vi "WHD_VEten_0.1.5.WS_BIDIR_Inycom_baja_velocidad.vi"() -> ()   [LabVIEW 2015]
uses:
  <vilib>/LabVIEW Targets/FPGA/cRIO/shared/nicrio_ModuleControls/nicrio_cRIO-9234_DataRatesRing2.ctl
  <vilib>/RTwatchdog.llb/Watchdog expiration actions.ctl
  <vilib>/userdefined/High Color/nirio_resource_hc.ctl
  <vilib>/Platform/TimedLoop/XDataNode/timing_clust.ctl
  <vilib>/Platform/TimedLoop/XDataNode/nitl_modes.ctl
  <vilib>/Platform/TimedLoop/XDataNode/wakeup.ctl
  <vilib>/Analysis/5stat.llb/RMS (DBL).vi
  <vilib>/FPGAPlugInAG/cRIO-9031/niLvFpga_Open_cRIO-9031.vi
  <vilib>/Utility/error.llb/Error Cluster From Error Code.vi
  <vilib>/rvi/errors/niLvFpgaAdjustHostInterfaceError.vi
  <vilib>/FPGAPlugInAG/cRIO-9031/niLvFpga_Run_cRIO-9031.vi
  <vilib>/rvi/interface/common/niFpgaWaitOnOcc.vi
  <vilib>/Utility/file.llb/Write Delimited Spreadsheet (string).vi
  <vilib>/FPGAPlugInAG/cRIO-9031/niLvFpga_Reset_cRIO-9031.vi
  <vilib>/measure/madcrms.llb/Basic Averaged DC-RMS for 1 Chan.vi
  <vilib>/measure/maspectr.llb/FFT Spectrum (Mag-Phase) for 1 Chan.vi
  <vilib>/Utility/config.llb/Write Key (Double).vi
  <vilib>/FPGAPlugInAG/cRIO-9031/niLvFpga_Close_cRIO-9031.vi
  <vilib>/rvi/interface/nirviOpenFPGA/nirviOpenFPGA.xnode
  FPGA Bitfiles/WRDArabia_FPGATarget_FPGA8a2wsBIdirec_ph5KjwleieA.lvbitx
  <vilib>/rvi/interface/nirviReadWriteControl/nirviReadWriteControl.xnode
  <vilib>/rvi/interface/nirviMethod/nirviMethod.xnode
  <vilib>/platform/TimedLoop/XDataNode/XDataNode.xnode
  <vilib>/rvi/interface/nirviCloseFPGA/nirviCloseFPGA.xnode
  <vilib>/NI_Real-Time Target Support.lvlib
  <vilib>/rvi/errors/niLvFpgaMergeErrorWithErrorCode.vi
  AURA_Wheel/Json2Labv.lvlib
  AURA_Wheel/AuraWheelAPI/AuraWheel.lvlib
  NiFpgaLv.dll
  <vilib>/FPGAPlugInAG/cRIO-9031/niLvFpga_ConfigureFifo_cRIO-9031.vi
  <vilib>/FPGAPlugInAG/cRIO-9031/niLvFpga_StartFifo_cRIO-9031.vi
  <vilib>/FPGAPlugInAG/cRIO-9031/niLvFpga_ReadFifo_cRIO-9031.vi
  <vilib>/FPGAPlugInAG/cRIO-9031/niLvFpga_StopFifo_cRIO-9031.vi
  <vilib>/measure/NI_MAPro.lvlib
  <vilib>/Analysis/NI_AALPro.lvlib
  <vilib>/Analysis/NI_AALBase.lvlib
  <vilib>/Utility/config.llb/NI_LVConfig.lvlib
  <vilib>/Platform/TimedLoop/XDataNode/XDNodeRunTimeDep.lvlib
  Library/IF2_Reader/IF2_Reader.lvlib
panel:
  out "size(s) 2":i32[](array[numeric])
  out "freq_cutlow":dbl
  out "freq_cuthigh":dbl
  out "Radios_por_ejes":dbl[](array[numeric])
  out "Radios ruedas":dbl[](array[numeric])
  out "Frequency":dbl[](array[numeric])
  out "Value to compare":dbl[](array[numeric])
  in  "Developer password":string
  out "Waveform Graph":waveform(sgl)[](graph)
  out "min":dbl[](array[numeric])
  out "max":dbl[](array[numeric])
  out "median":dbl[](array[numeric])
  out "mean":dbl[](array[numeric])
  in  "Accelerometer":i32
  out "Low cutoff freq":dbl
  out "noise_range":dbl
  out "Numeric":i32
  out "Calibration parameter":dbl
  out "Accel.detected":i32
  out "Mean\nfrequency":dbl format="%0.2f"
  out "Nº meas":i32
  out "Array":i32[](array[numeric])
  out "sorted array":i32[](array[numeric])
  out "Array 3":i32[](array[numeric])
  out "max value":i32
  out "max index(es)":i32
  out "element":i32
  out "size(s) 3":i32
  out "size(s)":i32[](array[numeric])
  out "Valid\nindex":i32[](array[numeric])
  out "Acquiring time":dbl
  out "Inicio pasada 2":timestamp
  out "calibration log":path
  out "date/time string 2":string
  out "Folder":path
  in  "Developer commad":string
  out "Save calibration":bool
  out "Pattern amplitude (g)":dbl=1.02
  out "Pattern frequency (Hz)":dbl=159.2
  out "Report":string
  out "AURA wheel test":bool
  out "LOG.txt":path
  out "Report_AURA":string
  out "error FPGA":errorcluster
  out "error AURA":errorcluster
  out "error manipulacion archivos":errorcluster
  out "Response headers":string
  out "Max RMS Ruedas":dbl[][](array[numeric])
  out "TAGs LR6":string[](array[string])
  out "TAGs HEX":string[](array[string])
  out "Parar":bool
  out "result":bool
  out "TAGs":string[](array[string])
  out "Temperatura (ºC)":dbl
  out "V (m/s)":dbl
  out "Digital?":bool=TRUE
  out "Watchdog config":T1={"reset"=FALSE, "occurrence"=FALSE, "trigger protocol"=enum."active high", "trigger line"=enum."none", "disable watchdog on VI exit"=TRUE}
  out "Tiempo de adquisicion":dbl=10.0
  out "Adquirir":bool
  out "Nº Ruedas 1":i32
  out "NºRuedas 2":i32
  out "Disco Duro Disponible (bytes)":i64
  out "Buffer Overflow":bool
  out "Buffer Underflow":bool
  out "Archivo\nvalido?":bool
  out "Número de ejes detectados":i32
  out "Ejes_convoy":i32
  out "Tiempo de paso (s)":dbl
  out "created path":path
  out "Nombre de archivo":path[](array[path])
  out "LR6 IP address":string="192.168.106.94"
  out "Port LR6":u16=2001
  out "T fuera rango":bool
  out "Frecuencia de muestreo (Hz)":dbl=25600.0
  out "Escaneos de la FIFO por canal":u32=5000
  out "Tiempo extra al detector de paso (s)":dbl=1.0
  out "dt RMS":dbl=256.0
  out "Frecuencia de muestreo y módulo CRIO":T2=2 items=["51.200 kS/s (NI 9234)"=1, "25.600 kS/s (NI 9234)"=2, "17.067 kS/s (NI 9234)"=3, "12.800 kS/s (NI 9234)"=4, "10.240 kS/s (NI 9234)"=5, "8.533 kS/s (NI 9234)"=6, "7.314 kS/s (NI 9234)"=7, "6.400 kS/s (NI 9234)"=8, "5.689 kS/s (NI 9234)"=9, "5.120 kS/s (NI 9234)"=10, "4.654 kS/s (NI 9234)"=11, "4.267 kS/s (NI 9234)"=12, "3.938 kS/s (NI 9234)"=13, "3.657 kS/s (NI 9234)"=14, "3.413 kS/s (NI 9234)"=15, "3.200 kS/s (NI 9234)"=16, "3.012 kS/s (NI 9234)"=17, "2.845 kS/s (NI 9234)"=18, "2.695 kS/s (NI 9234)"=19, "2.560 kS/s (NI 9234)"=20, "2.438 kS/s (NI 9234)"=21, "2.328 kS/s (NI 9234)"=22, "2.226 kS/s (NI 9234)"=23, "2.133 kS/s (NI 9234)"=24, "2.048 kS/s (NI 9234)"=25, "1.969 kS/s (NI 9234)"=26, "1.896 kS/s (NI 9234)"=27, "1.829 kS/s (NI 9234)"=28, "1.765 kS/s (NI 9234)"=29, "1.707 kS/s (NI 9234)"=30, "1.652 kS/s (NI 9234)"=31]
  out "Puerto RFID":u16=2189
  out "IP RFID":string="192.168.106.99"
  out "Offset_rueda WS 2":fxp<+/-,24,-4>=0.004999998956918716 format="%.27g"
  out "Count(mSec)":u32=2
  out "RFID NEM on?":bool
  out "RFID LR6 on?":bool
  out "Canal cero WS1?":bool
  out "Canal cero WS2":bool
  in  "Calibration":bool
  out "Direccion 0?":bool
  out "Boton Adquirir?":bool
  out "RuedaDetectada2?":bool=TRUE
  out "RuedaDetectada1?":bool=TRUE
  out "Timeout ruedas":dbl
  out "Borrar archivos\nadquisicion con error":bool
  out "Able watchdog?":bool
  out "Reset watchdog?":bool
  out "Leer config RFID NEM":bool
  out "bytes to read":i32
  out "DeviceAddress":u8
  out "timeout ms (60000)":i32
  out "Max archivos":u32=2
  out "Bytes libre despues de borrar":u32=2
  out "Bytes min libre":u32=2
  out "Nº de acelerómetros":i32
  out "Nº inductivos":i32
  out "Offset_rueda WS 1":fxp<+/-,24,-4>=0.004999998956918716 format="%.27g"
  out "TAGs_AURAwheel":string[][](array[string])
  out "Plataformas?":bool
  out "Nº Ejes":i32[](array[numeric])
  out "Nº UTs":i32
  out "it-read-LR6":i32[](array[numeric])
  out "it-LR6":i32
  out "RFID_LR6_Error":errorcluster
  out "Series_flota":string[](array[string])
  out "Tabla_flota":string[][](array[string])
  out "Puntos medios de las ventanas":dbl[][](array[numeric])
  out "configuration file path":path=path "c:/Parametros.cfg"
  out "IP synchr":string
  out "data":cluster{"status":string}
  out "confRFID":path=path "c:/RFID/TAGS.csv"
  out "TAGS leidos":path=path "c:/RFID/TAGS.csv"
  out "Use Aura?":bool
  out "Parametros AuraWheel":string[](array[string])
  out "Parámetros acelerómetros":dbl[](array[numeric])
  out "Fin":bool
  out "Contador":i32=1
  out "Path LOG":path=path "c:/TEST"
  out "Fallo fotocelula":bool
  out "Path_Borrar":path=path "c:/Trenes"
  out "Longitud de la unidad":dbl
  out "Aviso no detección":string
  out "Time to Acquire Block (ms)":i32
  out "Distancia de acelerómetros":dbl[](array[numeric])
  out "Block Size":u32
  out "Distancias generales":dbl[](array[numeric])
  out "Reset del controlador":bool
  out "Parar la aplicación":bool
  out "date/time string":string
  out "Timeout ruedas":bool
  out "Tiempo":dbl
  out "Inicio pasada":timestamp
  out "Ultimo TEST":timestamp
  out "Fuente":bool=TRUE
  out "DC OK":string
  out "Aviso temperatura":string
  out "connection ID":refnum<k5>
  # "Calibration - Noise analysis"
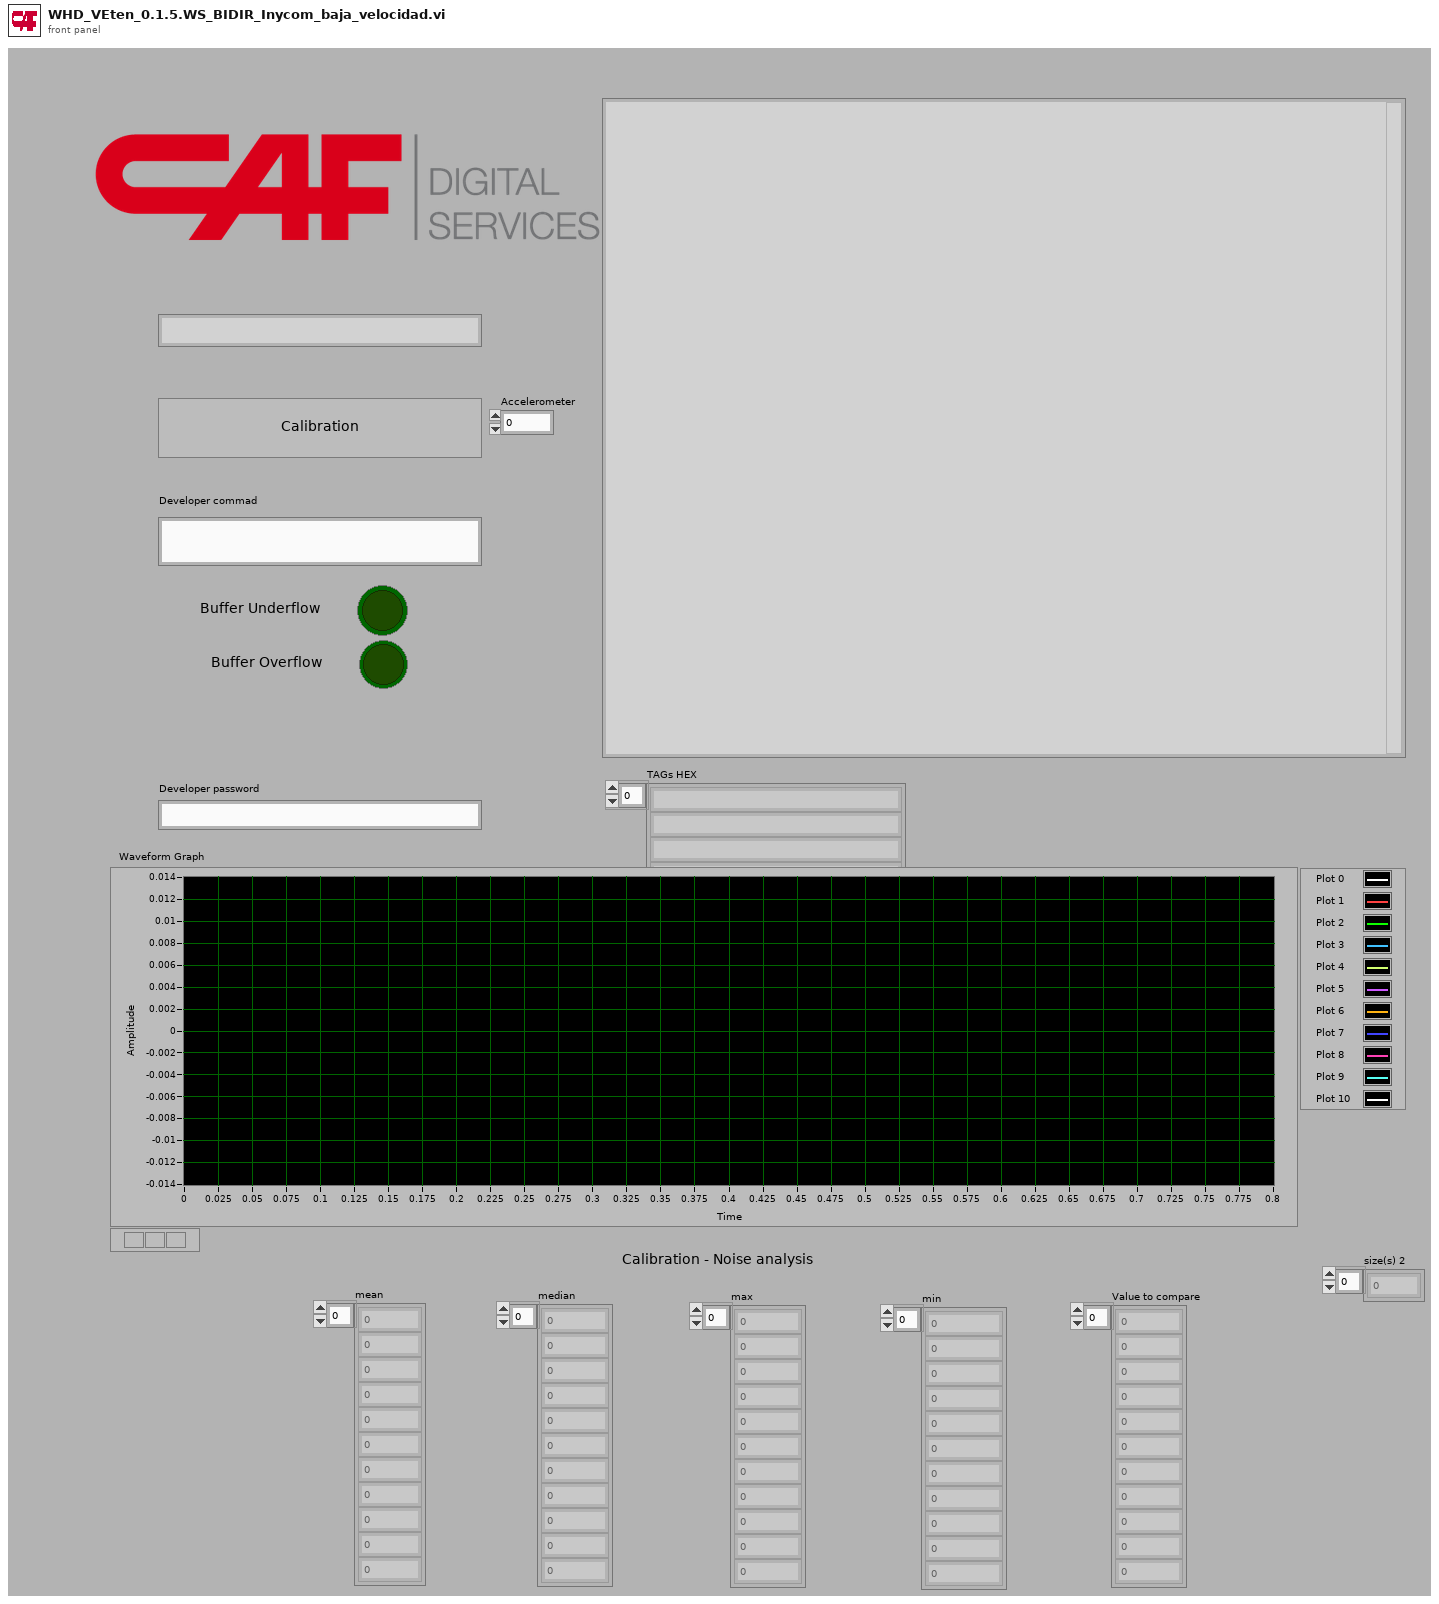
[diagram p1: front panel]
types:
  T1 = typedef "Watchdog expiration actions.ctl" = cluster{"reset":bool, "occurrence":bool, "trigger protocol":enum16{"active high", "active low", "open collector"}, "trigger line":enum16{"none", "line 0", "line 1", "line 2", "line 3", "line 4", "line 5", "line 6", "line 7", "SMB line 0"}, "disable watchdog on VI exit":bool}
  T2 = typedef "nicrio_cRIO-9234_DataRatesRing2.ctl" = u8
  T3 = typedef "nirio_resource_hc.ctl" = tag
  T4 = enum16{"open", "replace", "create", "open or create", "replace or create", "replace or create with confirmation"}
  T5 = enum16{"big-endian, network order", "native, host order", "little-endian"}
  T6 = typedef "XDNodeRunTimeDep.lvlib/timing_clust.ctl" = cluster{"Expected End [f-1]":u64, "Actual End [f-1]":u64, "Finished Late? [f-1]":bool, "Expected End [i-1]":u64, "Actual End [i-1]":u64, "Finished Late? [i-1]":bool, "Expected Start [i]":u64, "Actual Start [i]":u64, "Expected Start [f]":u64, "Actual Start [f]":u64, "Source Name":string, "Structure Name":string, "Period":i64, "Deadline":i64, "Offset":i64, "Start":i64, "Priority":i32, "Timeout":i32, "Mode":T7, "Wakeup Reason":T8, "Error":errorcluster, "Source Type":string, "Secondary Source Type":string, "Global End Time":u64, "Global Start Time":u64, "Frame Duration":u64, "Iteration Duration":u64, "Assigned CPU":i32, "I/O Scan Engine Mode":u32}
  T7 = typedef "XDNodeRunTimeDep.lvlib/nitl_modes.ctl" = enum32{"No Change", "Process missed periods, maintain original phase", "Discard missed periods, maintain original phase", "Process missed periods, ignore original phase", "Discard missed periods, ignore original phase"}
  T8 = typedef "XDNodeRunTimeDep.lvlib/wakeup.ctl" = enum32{"Normal", "Aborted", "Asynchronous wakeup", "Timing source error", "Timed loop error", "Timeout"}
  T9 = cluster{"error IO":errorcluster, bool[], u32[], string[], dbl[]}
  T10 = cluster{"error out":errorcluster, dbl[], "TagArray":string[], "Direccion 0?":bool}
  T11 = cluster{"g_ts":dbl, "p_sp":dbl, "p_tp":dbl, "p_tg":cluster{"tg_n":dbl, "tg_t":string}[], "p_ax":cluster{"ax_n":dbl, "ax_sp":dbl, "ax_wh":cluster{"wh_p":dbl, "wh_a1":dbl, "wh_a2":dbl, "wh_a3":dbl, "wh_a4":dbl}[], "ax_fq":cluster{"wh_p":dbl, "wh_a1":dbl, "wh_a2":dbl, "wh_a3":dbl, "wh_a4":dbl}[], "ax_amp":cluster{"wh_p":dbl, "wh_a1":dbl, "wh_a2":dbl, "wh_a3":dbl, "wh_a4":dbl}[], "ax_en":cluster{"wh_p":dbl, "wh_a1":dbl, "wh_a2":dbl, "wh_a3":dbl, "wh_a4":dbl}[]}[]}
  T12 = typedef "NI_LVConfig.lvlib/Config Data RefNum.ctl" = refnum<k1>
  T13 = cluster{"IP":string, "Port":u16, "ReaderConfigFile":path, "ROspecConfigFile":path}
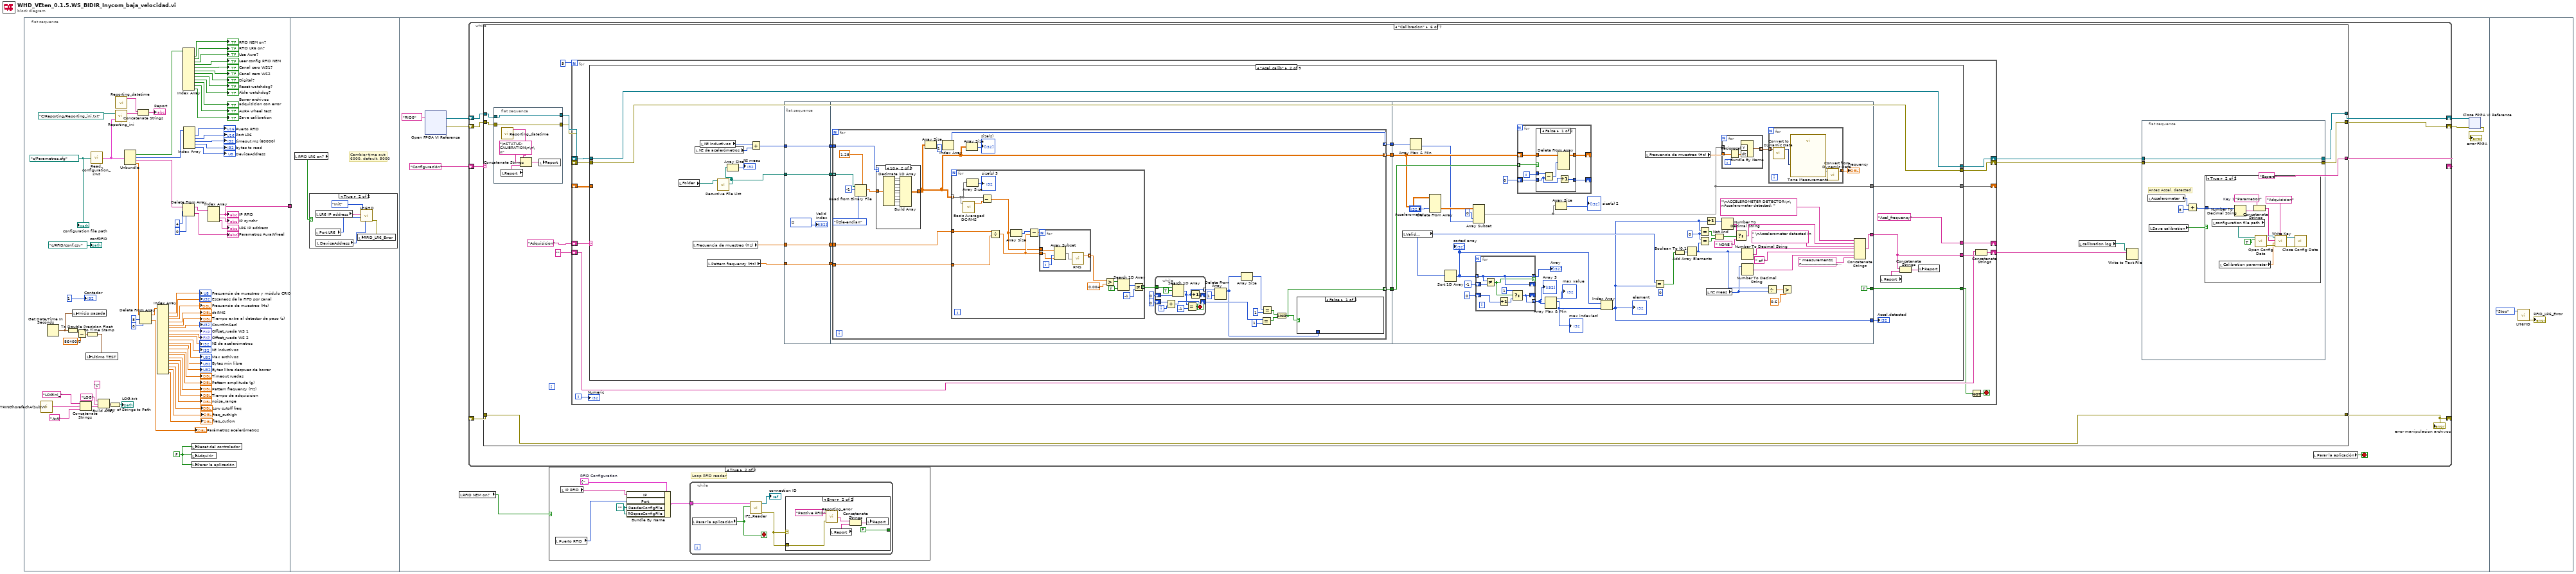
[diagram p0: block diagram]
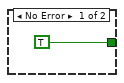
[diagram p4: hidden frame]
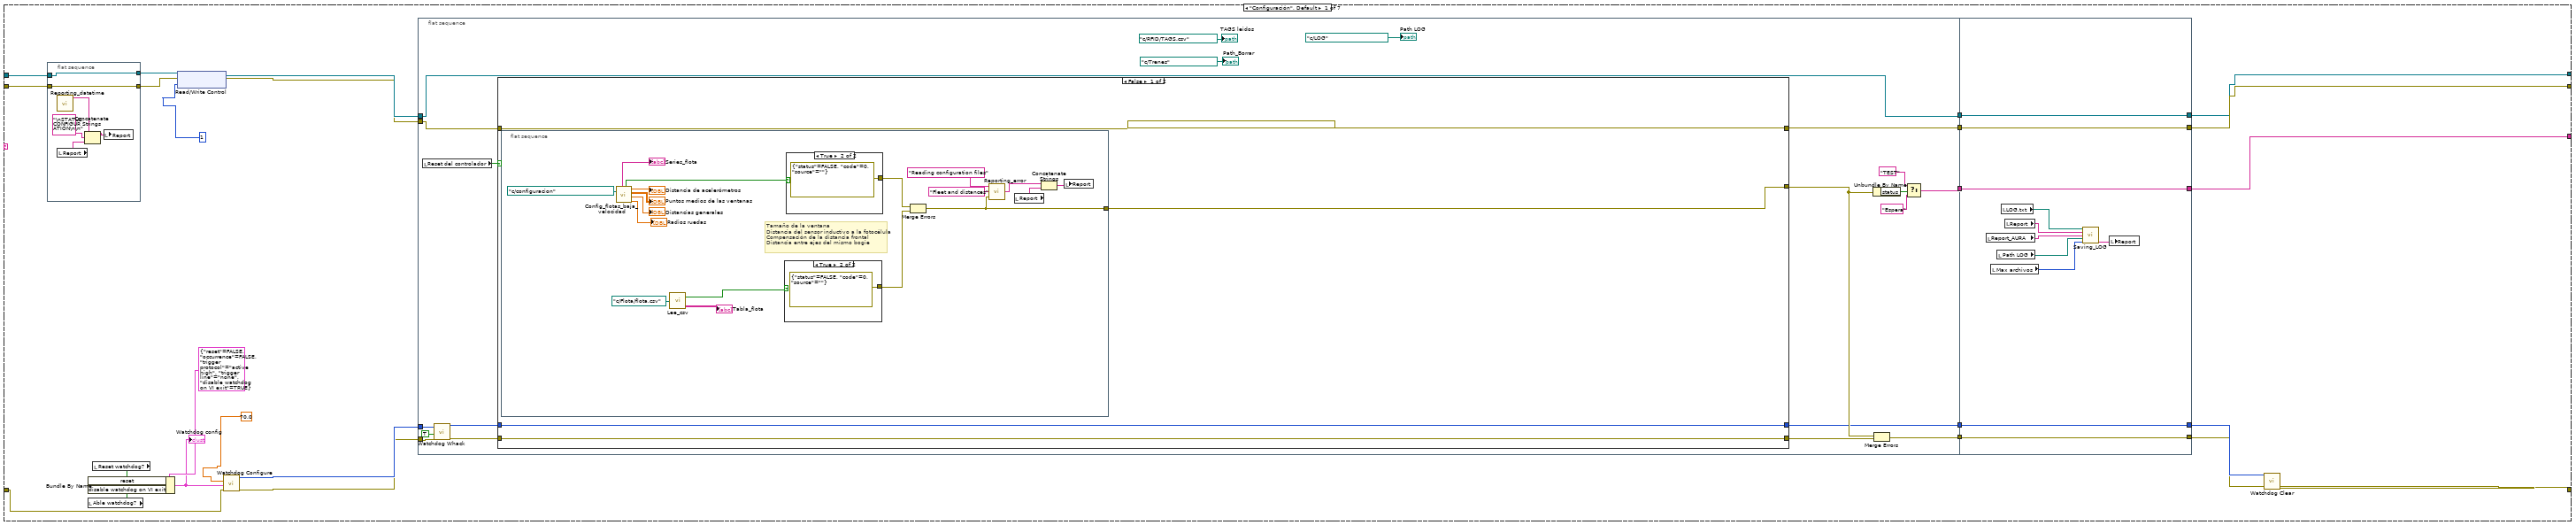
[diagram p5: hidden frame]
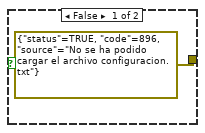
[diagram p6: hidden frame]
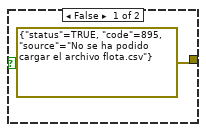
[diagram p7: hidden frame]
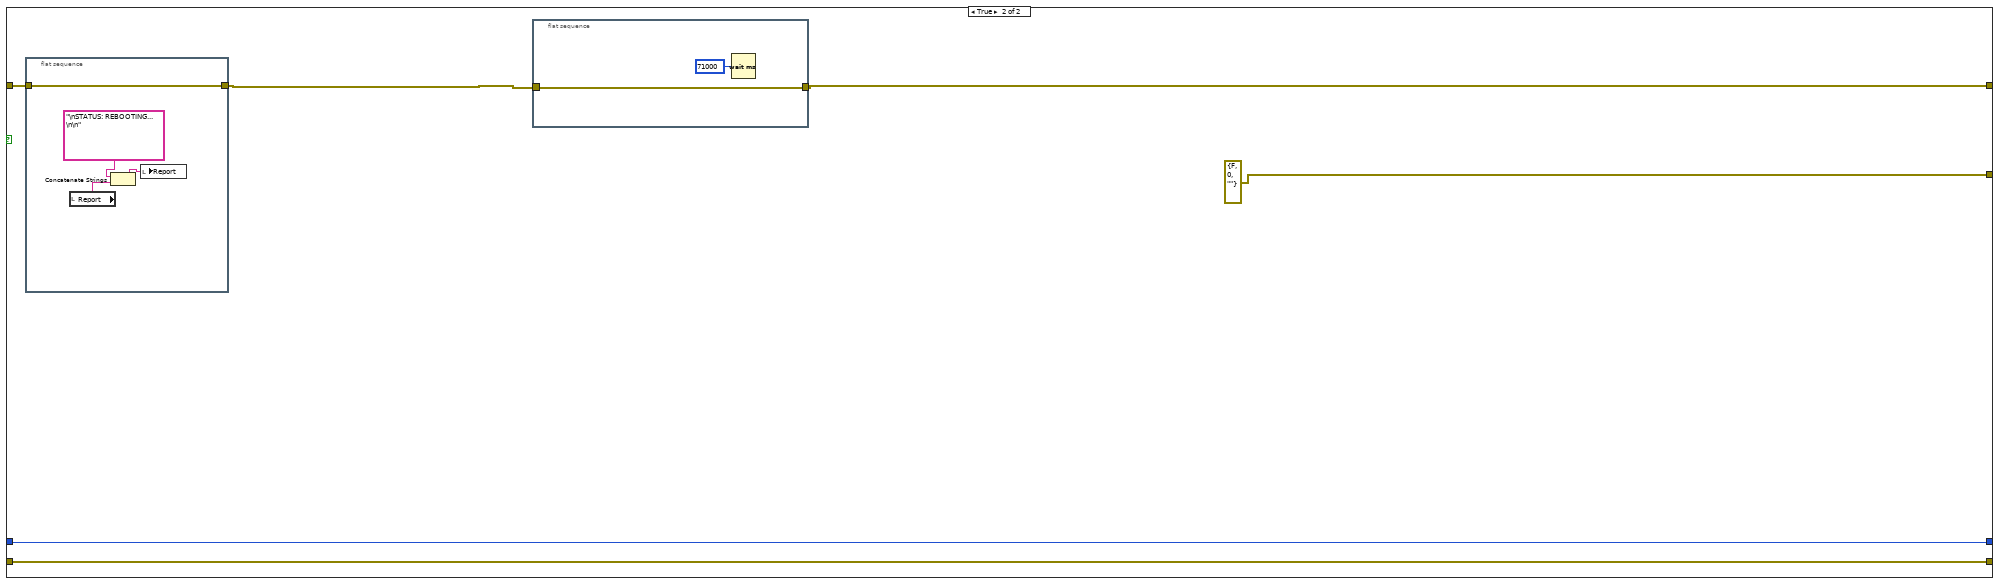
[diagram p8: hidden frame]
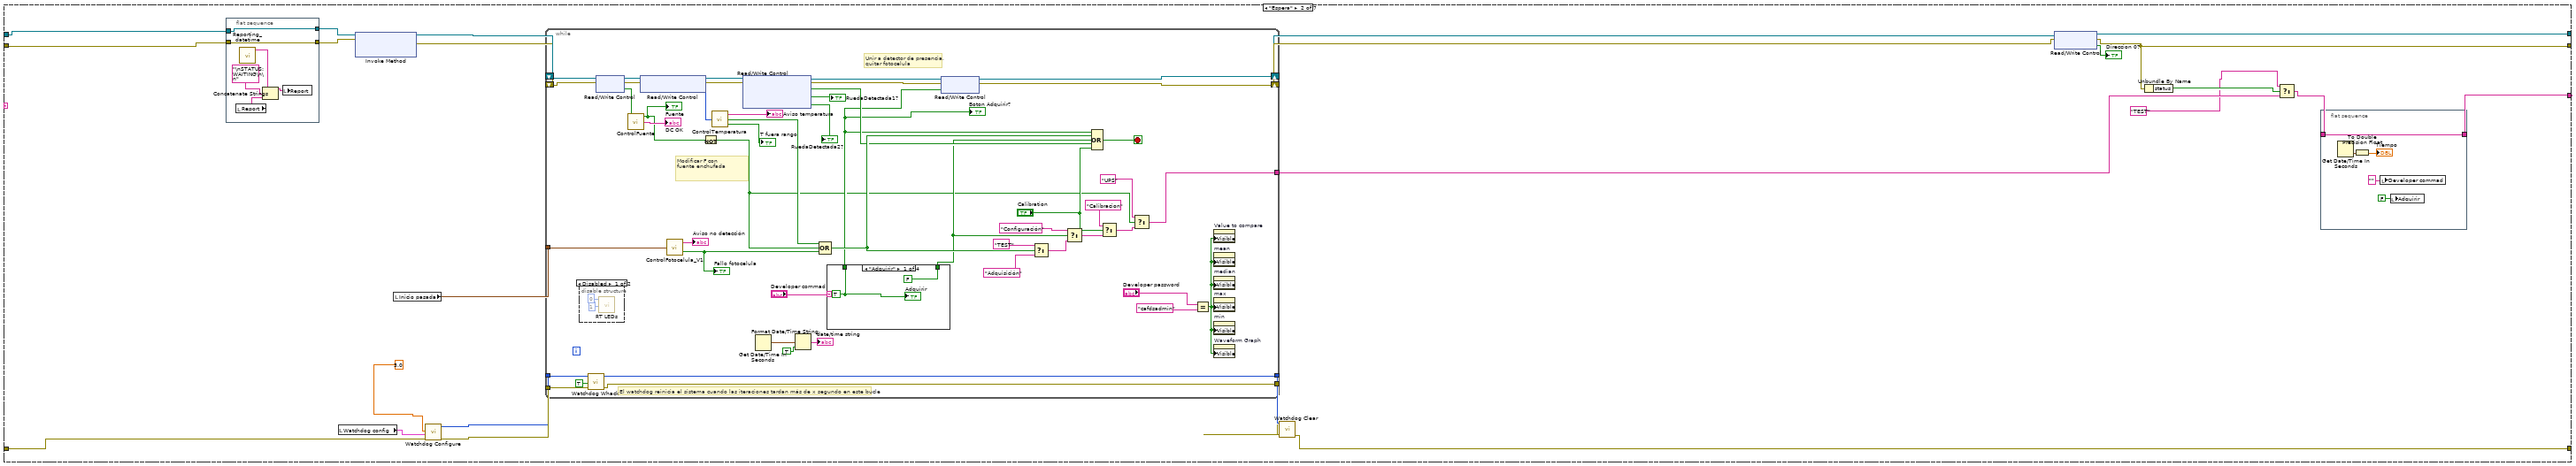
[diagram p9: hidden frame]
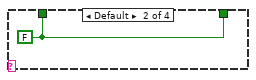
[diagram p10: hidden frame]
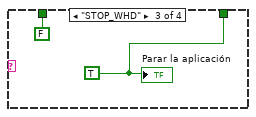
[diagram p11: hidden frame]
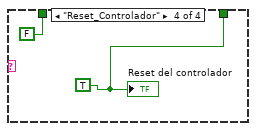
[diagram p12: hidden frame]
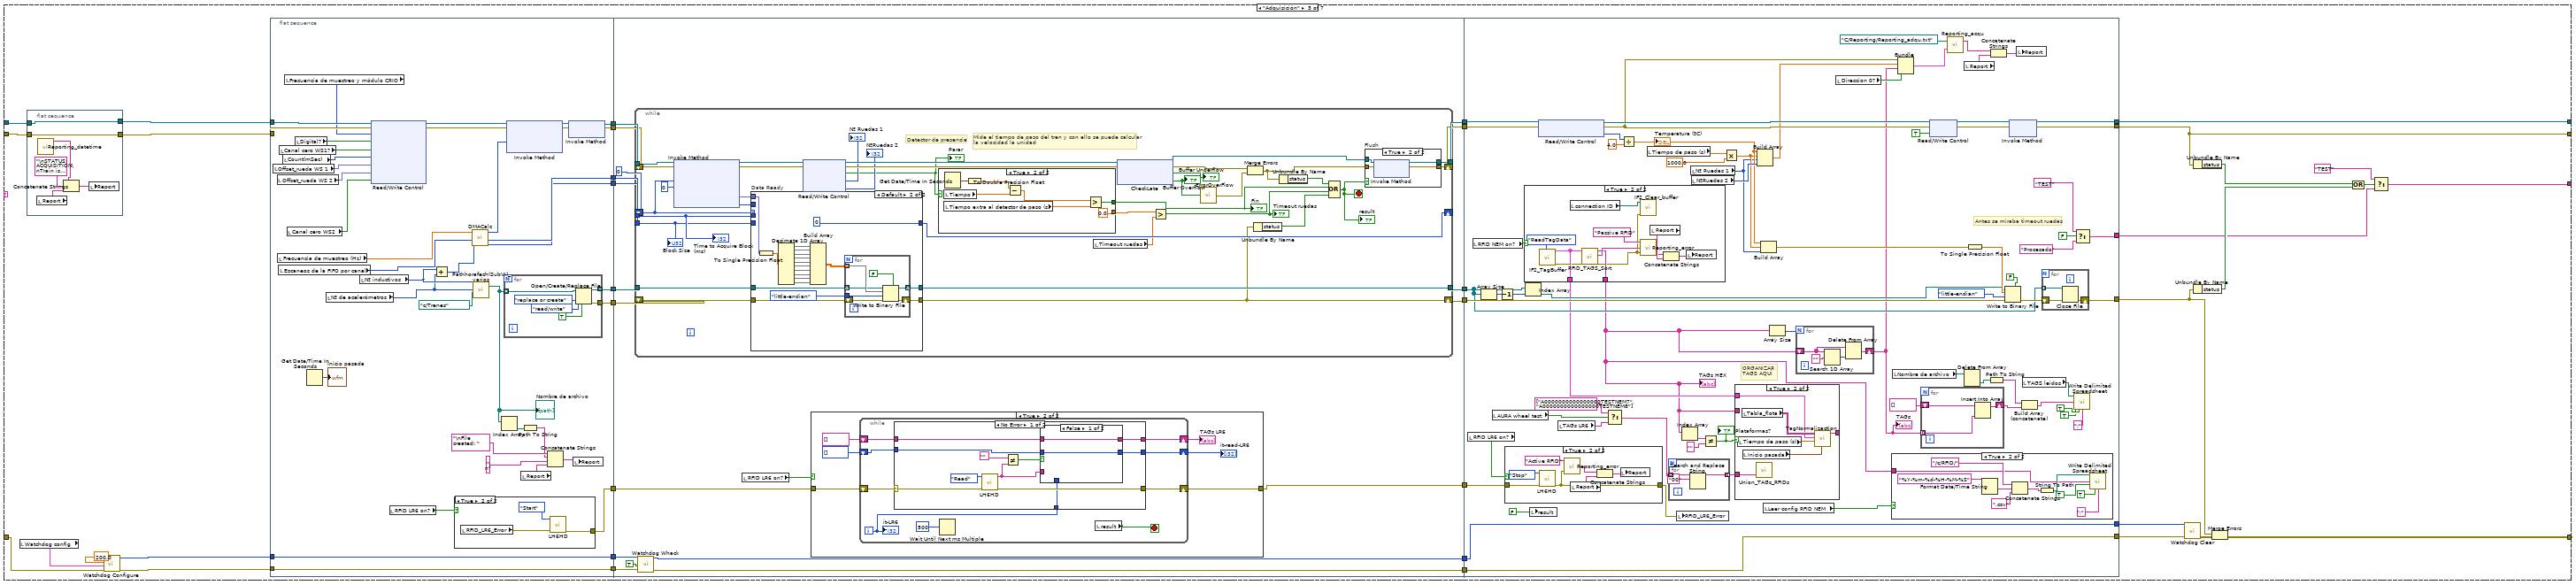
[diagram p14: hidden frame]
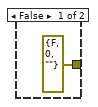
[diagram p15: hidden frame]
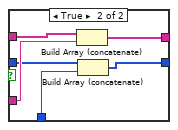
[diagram p17: hidden frame]
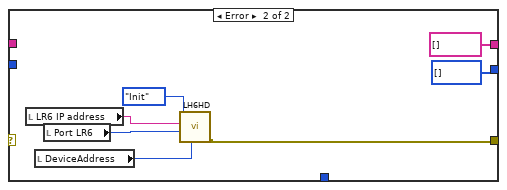
[diagram p18: hidden frame]
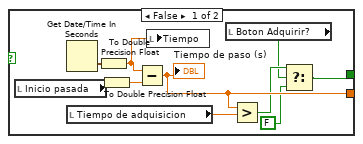
[diagram p19: hidden frame]
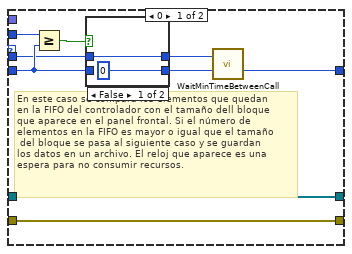
[diagram p20: hidden frame]
diagram:
  n1 = flat-sequence {
    tunnel: [w6] -> w1
    tunnel: w1 -> [_]
    frame #0 {
      w7 = FALSE ("Reset del controlador")
      w68 = path "c:/Parametros.cfg" ("configuration file path")
      n2 = call "STRINGhorafechA(SubVI).vi"() -> ("STRINGhora_fecha"=w18:string)
      n3 = Get Date/Time In Seconds() -> (seconds since 1Jan1904=w73:timestamp)
      n4 = To Double Precision Float(number=w73) -> (double precision float=w75:dbl)
      n5 = local write "Inicio pasada"(w73) -> ()
      n6 = Subtract(x=w75, y=86400.0) -> (x-y=w74:dbl)
      n7 = Concatenate Strings("LOGini_" ("string"), w18, ".txt" ("string")) -> (w20:string)
      n8 = To Time Stamp(1:w74) -> (0:w72:timestamp)
      n9 = local write "Ultimo TEST"(w72) -> ()
      n10 = call "Read_configuration_2ws.vi"("configuration file path"=w68) -> ("output cluster"=w24:T9)
      n11 = Build Array("c", "LOG" ("element"), w20) -> (w17:string[])
      n12 = Array of Strings to Path(0:w17) -> (2:→"LOG.txt":path)  [unwired: 1 out]
      n13 = call "Reporting_ini.vi"("Configuration cluster"=w24, "address repoting"=path "C:/Reporting/Reporting_ini.txt" ("file (use dialog)")) -> ("Reporting"=w23:string)  [unwired: 1 in]
      n14 = call "Reporting_datetime.vi"() -> ("String"=w21:string)  [unwired: 11 in]
      n15 = Unbundle(w24) -> (w71:bool[], w70:u32[], w63:string[], w67:dbl[])  [unwired: 1 out]
      n16 = Concatenate Strings(w21, w23) -> (→"Report":string)
      n17 = Delete From Array(array=w67, length=8, index=8) -> (deleted portion=→"Parámetros acelerómetros":dbl[], array with subset deleted=w66:dbl[])
      n18 = Index Array(array=w66) -> (element #1=→"Frecuencia de muestreo y módulo CRIO":dbl, element #2=→"Escaneos de la FIFO por canal":dbl, element #3=→"Frecuencia de muestreo (Hz)":dbl, element #4=→"dt RMS":dbl, element #5=→"Tiempo extra al detector de paso (s)":dbl, element #6=→"Count(mSec)":dbl, element #7=→"Offset_rueda WS 1":dbl, element #8=→"Offset_rueda WS 2":dbl, element #9=→"Nº de acelerómetros":dbl, element #10=→"Nº inductivos":dbl, element #11=→"Max archivos":dbl, element #12=→"Bytes min libre":dbl, element #13=→"Bytes libre despues de borrar":dbl, element #14=→"Timeout ruedas":dbl, element #15=→"Pattern amplitude (g)":dbl, element #16=→"Pattern frequency (Hz)":dbl, element #17=→"Tiempo de adquisicion":dbl, element #18=→"noise_range":dbl, element #19=→"Low cutoff freq":dbl, element #20=→"freq_cuthigh":dbl, element #21=→"freq_cutlow":dbl)  [unwired: 21 in]
      n19 = Index Array(array=w71) -> (element #1=→"RFID NEM on?":bool, element #2=→"RFID LR6 on?":bool, element #3=→"Use Aura?":bool, element #4=→"Leer config RFID NEM":bool, element #5=→"Canal cero WS1?":bool, element #6=→"Canal cero WS2":bool, element #7=→"Digital?":bool, element #8=→"Reset watchdog?":bool, element #9=→"Able watchdog?":bool, element #10=→"Borrar archivos\nadquisicion con error":bool, element #11=→"AURA wheel test":bool, element #12=→"Save calibration":bool)  [unwired: 12 in]
      n20 = Delete From Array(array=w63, length=4, index=0) -> (deleted portion=→"Parametros AuraWheel":string[], array with subset deleted=w62:string[])
      n21 = Index Array(array=w70) -> (element #1=→"Puerto RFID":u32, element #2=→"Port LR6":u32, element #3=→"timeout ms (60000)":u32, element #4=→"bytes to read":u32, element #5=→"DeviceAddress":u32)  [unwired: 5 in]
      n22 = local write "Reset del controlador"(w7) -> ()
      n23 = local write "Adquirir"(w7) -> ()
      n24 = local write "Parar la aplicación"(w7) -> ()
      n25 = Index Array(array=w62) -> (element #1=w6:string, element #2=→"IP synchr":string, element #3=→"LR6 IP address":string)  [unwired: 3 in]
      "IP RFID" <- w6
      "Contador" <- 1
      "confRFID" <- path "c:/RFID/conf.csv" ("file path (use dialog)")
      "configuration file path" <- w68
    }
    frame #1 {
      # "Cambiar time out:\n6000, default, 5000"
      n26 = local read "RFID LR6 on?"() -> (w77:bool)
      n27 = case shown="True" w77 {
        frame False {
        }
        frame True {
          n28 = local read "LR6 IP address"() -> (w78:string)
          n29 = local read "Port LR6"() -> (w79:u16)
          n30 = local read "DeviceAddress"() -> (w80:u8)
          n31 = call "LH6HD.vi"("DeviceAddress"=w80, "Reader Port"=w79, "IP Address"=w78, "Action"=enum16{"Init", "Start", "Read", "Stop", "Exit"}."Init") -> ("error out"=w82:errorcluster)  [unwired: 6 in, 1 out]
          n32 = local write "RFID_LR6_Error"(w82) -> ()
        }
      }
    }
    frame #2 {
      n33 = xnode "Open FPGA VI Reference"("resource name"=T3 "RIO0") -> ("FPGA VI Reference Out"=w90:refnum<k20>, "error out"=w89:errorcluster)  [unwired: 1 in]
      n34 = local read "RFID NEM on?"() -> (w83:bool)
      n35 = while {
        shift-right: [w107] -> _
        shift-left: "Configuración" -> [w115]
        shift-right: [w109] -> w86
        shift-left: w90 -> [w114]
        shift-right: [w108] -> w85
        shift-left: w89 -> [w113]
        shift-right: [w112] -> _
        shift-left: _ -> [w111]
        stop <- w110 stop-if-true
        n36 = case shown="\"Calibracion\"" w115 {
          tunnel: [w130 w234 w329 w695 w983 "Espera" "Espera" ("t")] -> w107
          tunnel: [w140 w222 w343 w684 w982 w1049 w1843] -> w109
          tunnel: [w141 w221 w344 w682 w981 w1047 w1842] -> w108
          tunnel: w114 -> [w124 w220 w315 w685 w982 w1060 w1837]
          tunnel: w113 -> [w123 w219 w314 w683 w974 w1059 w1839]
          tunnel: [w137 w228 w341 w680 w973 w1048 w1840] -> w112
          tunnel: w111 -> [w129 w233 w325 w694 w970 w1048 w1840]
          frame "Configuración", Default {
            n37 = flat-sequence {
              tunnel: w124 -> [w147]
              tunnel: w123 -> [w146]
              tunnel: [w147] -> w122
              tunnel: [w146] -> w121
              frame #0 {
                n38 = call "Reporting_datetime.vi"() -> ("String"=w142:string)  [unwired: 11 in]
                n39 = local read "Report"() -> (w143:string)
                n40 = Concatenate Strings(w142, "\nSTATUS: CONFIGURATION\n\n", w143) -> (w145:string)
                n41 = local write "Report"(w145) -> ()
              }
            }
            n42 = local read "Able watchdog?"() -> (w134:bool)
            n43 = local read "Reset watchdog?"() -> (w135:bool)
            n44 = Bundle By Name(cluster=T1 {"reset"=FALSE, "occurrence"=FALSE, "trigger protocol"=enum."active high", "trigger line"=enum."none", "disable watchdog on VI exit"=TRUE} ("expiration actions"), "reset"=w135, "disable watchdog on VI exit"=w134) -> (w128:T1)
            "Watchdog config" <- w128
            n45 = xnode "Read/Write Control"("FPGA VI Reference In"=w122, "error in"=w121, "Cycles to Filter"=u16 1) -> ("FPGA VI Reference Out"=w133:refnum<k20>, "error out"=w132:errorcluster)
            n46 = call <vilib>:"Watchdog Configure.vi"("error in (no error)"=w129, "expiration actions"=w128, "timeout (1 sec)"=70.0) -> ("error out"=w125:errorcluster, "watchdogID"=w126:u64)  [unwired: 1 in, 2 out]
            n47 = flat-sequence {
              tunnel: w133 -> [w159]
              tunnel: w132 -> [w156]
              tunnel: w126 -> [w149]
              tunnel: w125 -> [w148]
              tunnel: [w158] -> w120
              tunnel: [w166] -> w119
              tunnel: [w159] -> w118
              tunnel: [w161] -> w117
              tunnel: [w153] -> w116
              tunnel: [w212] -> w139
              tunnel: [w213] -> w138
              tunnel: [w214] -> w140
              tunnel: [w215] -> w130
              tunnel: [w216] -> w141
              tunnel: w120 -> [w216]
              tunnel: w119 -> [w215]
              tunnel: w118 -> [w214]
              tunnel: w117 -> [w213]
              tunnel: w116 -> [w212]
              frame #0 {
                n48 = local read "Reset del controlador"() -> (w155:bool)
                n49 = call <vilib>:"Watchdog Whack.vi"("error in (no error)"=w148, "reset watchdog after expire? (F)"=TRUE, "watchdogID in"=w149) -> ("error out"=w151:errorcluster, "watchdogID out"=w152:u64)  [unwired: 2 in, 1 out]
                n50 = case shown="False" w155 {
                  tunnel: w156 -> [w171 w195]
                  tunnel: [w171 w198] -> w158
                  tunnel: [w168 errorcluster {"status"=FALSE, "code"=0, "source"=""} ("error IO")] -> w157
                  tunnel: [w170 w197] -> w153
                  tunnel: w152 -> [w170 w197]
                  tunnel: w151 -> [w169 w196]
                  tunnel: [w169 w196] -> w150
                  frame False {
                    n51 = flat-sequence {
                      tunnel: [w179] -> w168
                      frame #0 {
                        # "Tamaño de la ventana\nDistancia del sensor inductivo a la fotocélula\nCompensación de la distancia frontal\nDistancia entre ejes del mismo bogie"
                        n52 = call "Config_flotas_baja_velocidad.vi"("file path (dialog if empty)"=path "c:/configuracion") -> ("Radios ruedas"=→"Radios ruedas":dbl[], "Distancias generales"=→"Distancias generales":dbl[], "Puntos medios de las ventanas"=→"Puntos medios de las ventanas":dbl[][], "Distancia de acelerómetros"=→"Distancia de acelerómetros":dbl[], "Distacias y medidas de dispositivos"=w176:bool, "Series_flota"=→"Series_flota":string[])  [unwired: 5 in]
                        n53 = call "Lee_csv.vi"("Path"=path "c:/Flota/flota.csv") -> ("Tabla_flota"=→"Tabla_flota":string[][], "Lectura_OK?"=w187:bool)
                        n54 = case shown="True" w187 {
                          tunnel: [errorcluster {"status"=TRUE, "code"=895, "source"="No se ha podido cargar el archivo flota.csv"} ("error out") errorcluster {"status"=FALSE, "code"=0, "source"=""} ("error out")] -> w188
                          frame False {
                          }
                          frame True {
                          }
                        }
                        n55 = case shown="True" w176 {
                          tunnel: [errorcluster {"status"=TRUE, "code"=896, "source"="No se ha podido cargar el archivo configuracion.txt"} ("error out") errorcluster {"status"=FALSE, "code"=0, "source"=""} ("error out")] -> w189
                          frame False {
                          }
                          frame True {
                          }
                        }
                        n56 = Merge Errors(w189, w188) -> (w179:errorcluster)
                        n57 = call "Reporting_error.vi"("error out 2"=w179, "Concept explanation"="Fleet and distances", "Concept"="Reading configuration files") -> ("Reporting"=w181:string)
                        n58 = local read "Report"() -> (w180:string)
                        n59 = Concatenate Strings(w181, w180) -> (w182:string)
                        n60 = local write "Report"(w182) -> ()
                      }
                    }
                  }
                  frame True {
                    n61 = flat-sequence {
                      tunnel: w195 -> [w203]
                      tunnel: [w203] -> w194
                      frame #0 {
                        n62 = local read "Report"() -> (w202:string)
                        n63 = Concatenate Strings("\nSTATUS: REBOOTING...\n\n", w202) -> (w200:string)
                        n64 = local write "Report"(w200) -> ()
                      }
                    }
                    n65 = flat-sequence {
                      tunnel: [w205] -> w198
                      tunnel: w194 -> [w205]
                      frame #0 {
                        n66 = Wait (ms)(milliseconds to wait=u32 71000) -> ()  [unwired: 1 out]
                      }
                    }
                  }
                }
                n67 = Unbundle By Name(w157) -> ("status"=w167:bool)
                n68 = Merge Errors(w157, w150) -> (w161:errorcluster)
                n69 = Select(t="TEST", s=w167, f="Espera") -> (s? t:f=w166:string)
                "Path_Borrar" <- path "c:/Trenes" ("file path (use dialog)")
                "Path LOG" <- path "c:/LOG" ("file path (use dialog)")
                "TAGS leidos" <- path "c:/RFID/TAGS.csv" ("file path (use dialog)")
              }
              frame #1 {
                n70 = local read "Report_AURA"() -> (w209:string)
                n71 = local read "Max archivos"() -> (w210:u32)
                n72 = local read "Path LOG"() -> (w211:path)
                n73 = local read "LOG.txt"() -> (w206:path)
                n74 = local read "Report"() -> (w208:string)
                n75 = call "Saving_LOG.vi"("Path"=w206, "Report"=w208, "Report AURA"=w209, "Path Carpeta"=w211, "Nº Archivos Max"=w210) -> ("Report"=w207:string)  [unwired: 9 in, 1 out]
                n76 = local write "Report"(w207) -> ()
              }
            }
            n77 = call <vilib>:"Watchdog Clear.vi"("error in (no error)"=w138, "watchdogID in"=w139) -> ("error out"=w137:errorcluster)  [unwired: 5 in]
          }
          frame "Espera" {
            n78 = flat-sequence {
              tunnel: w220 -> [w247]
              tunnel: w219 -> [w246]
              tunnel: [w247] -> w218
              tunnel: [w246] -> w217
              frame #0 {
                n79 = local read "Report"() -> (w243:string)
                n80 = call "Reporting_datetime.vi"() -> ("String"=w242:string)  [unwired: 11 in]
                n81 = Concatenate Strings(w242, "\nSTATUS: WAITING\n\n", w243) -> (w245:string)
                n82 = local write "Report"(w245) -> ()
              }
            }
            n83 = local read "Watchdog config"() -> (w227:T1)
            n84 = xnode "Invoke Method"("FPGA VI Reference In"=w218, "error in"=w217) -> ("FPGA VI Reference Out"=w237:refnum<k20>, "error out"=w236:errorcluster)  [unwired: 1 in]
            n85 = local read "Inicio pasada"() -> (w241:timestamp)
            n86 = call <vilib>:"Watchdog Configure.vi"("error in (no error)"=w233, "expiration actions"=w227, "timeout (1 sec)"=3.0) -> ("error out"=w232:errorcluster, "watchdogID"=w231:u64)  [unwired: 1 in, 2 out]
            n87 = while {
              tunnel: [w258] -> w240
              shift-right: [w274] -> w223
              shift-left: w237 -> [w282]
              shift-right: [w273] -> w224
              shift-left: w236 -> [w281]
              tunnel: w241 -> [w285]
              tunnel: w232 -> [w271]
              tunnel: w231 -> [w272]
              tunnel: [w270] -> w230
              tunnel: [w269] -> w229
              stop <- w264 stop-if-true
              # "Modificar F con\nfuente enchufada"
              # "Unir a detector de presencia,\nquitar fotocelula"
              # "El watchdog reinicia el sistema cuando las iteraciones tardan más de x segundo en este bucle"
              n88 = disable-structure shown="Disabled" {
                frame Disabled {
                  n89 = call <vilib>:"RT LEDs.vi"("State"=1, "LED Num"=0) -> ()  [unwired: 1 in, 5 out]
                }
                frame Enabled {
                }
              }
              n90 = call <vilib>:"Watchdog Whack.vi"("error in (no error)"=w271, "reset watchdog after expire? (F)"=TRUE, "watchdogID in"=w272) -> ("error out"=w269:errorcluster, "watchdogID out"=w270:u64)  [unwired: 2 in, 1 out]
              n91 = xnode "Read/Write Control"("FPGA VI Reference In"=w282, "error in"=w281) -> ("FPGA VI Reference Out"=w294:refnum<k20>, "error out"=w293:errorcluster, "DC OK"=w298:bool)
              n92 = call "ControlFuente.vi"("DC OK 3"=w298) -> ("DC OK 2"=w260:bool, "DC OK"=→"DC OK":string)  [unwired: 1 out]
              "Fuente" <- w260
              n93 = xnode "Read/Write Control"("FPGA VI Reference In"=w294, "error in"=w293) -> ("FPGA VI Reference Out"=w289:refnum<k20>, "error out"=w288:errorcluster, "Chassis Temperature"=w296:i16)
              n94 = call "ControlFotocelula_V1.vi"("Tiempo de entrada a espera"=w285) -> ("Aviso no detección"=→"Aviso no detección":string, "Boolean"=w286:bool)
              "Fallo fotocelula" <- w286
              n95 = Not(x=w260) -> (.not. x?=w256:bool)
              n96 = call "ControlTemperatura.vi"("Chassis Temperature"=w296) -> ("Aviso temperatura"=→"Aviso temperatura":string, "Boolean"=w290:bool, "T fuera rango"=→"T fuera rango":bool)
              n97 = xnode "Read/Write Control"("FPGA VI Reference In"=w289, "error in"=w288) -> ("FPGA VI Reference Out"=w284:refnum<k20>, "error out"=w283:errorcluster, "Detector de presencia"=w277:bool, "RuedaDetectada1?"=→"RuedaDetectada1?":bool, "RuedaDetectada2?"=→"RuedaDetectada2?":bool)
              n98 = Get Date/Time In Seconds() -> (seconds since 1Jan1904=w279:timestamp)
              n99 = Format Date/Time String(seconds (now)=w279, UTC format=TRUE) -> (date/time string=→"date/time string":string)  [unwired: 1 in]
              n100 = Compound Arithmetic op=OR(w290, w256, w286) -> (w287:bool)
              n101 = case shown="\"Adquirir\"" "Developer commad" {
                tunnel: [w304 w305 FALSE ("Adquirir") FALSE ("Adquirir")] -> w263
                tunnel: [FALSE ("Adquirir") w305 w306 w308] -> w262
                frame "Adquirir" {
                  w304 = TRUE ("Adquirir")
                  "Adquirir" <- w304
                }
                frame Default {
                  w305 = FALSE ("Adquirir")
                }
                frame "STOP_WHD" {
                  w306 = TRUE ("Adquirir")
                  "Parar la aplicación" <- w306
                }
                frame "Reset_Controlador" {
                  w308 = TRUE ("Adquirir")
                  "Reset del controlador" <- w308
                }
              }
              "Boton Adquirir?" <- w263
              n102 = xnode "Read/Write Control"("FPGA VI Reference In"=w284, "error in"=w283, "Fotocélula"=w263) -> ("FPGA VI Reference Out"=w274:refnum<k20>, "error out"=w273:errorcluster)
              n103 = Select(t="TEST", s=w287, f="Adquisición") -> (s? t:f=w299:string)
              n104 = Select(t="Configuración", s=w262, f=w299) -> (s? t:f=w267:string)
              n105 = Compound Arithmetic op=OR(w263, w287, w262, w277, "Calibration") -> (w264:bool)
              n106 = Select(t="Calibracion", s="Calibration", f=w267) -> (s? t:f=w259:string)
              n107 = Select(t="UPS", s=w256, f=w259) -> (s? t:f=w258:string)
              n108 = Equal?(x="Developer password", y="cafdsadmin") -> (x = y?=w253:bool)
              n109 = property on="Value to compare" class="Arr (strict)"("Visible"=w253) -> ()  [unwired: 2 in, 2 out]
              n110 = property on="mean" class="Arr (strict)"("Visible"=w253) -> ()  [unwired: 2 in, 2 out]
              n111 = property on="median" class="Arr (strict)"("Visible"=w253) -> ()  [unwired: 2 in, 2 out]
              n112 = property on="max" class="Arr (strict)"("Visible"=w253) -> ()  [unwired: 2 in, 2 out]
              n113 = property on="min" class="Arr (strict)"("Visible"=w253) -> ()  [unwired: 2 in, 2 out]
              n114 = property on="Waveform Graph" class="WFGraph (strict)"("Visible"=w253) -> ()  [unwired: 2 in, 2 out]
            }
            n115 = call <vilib>:"Watchdog Clear.vi"("error in (no error)"=w229, "watchdogID in"=w230) -> ("error out"=w228:errorcluster)  [unwired: 5 in]
            n116 = xnode "Read/Write Control"("FPGA VI Reference In"=w223, "error in"=w224) -> ("FPGA VI Reference Out"=w222:refnum<k20>, "error out"=w221:errorcluster, "Direccion 0?"=→"Direccion 0?":bool)
            n117 = Unbundle By Name(w221) -> ("status"=w239:bool)
            n118 = Select(t="TEST", s=w239, f=w240) -> (s? t:f=w235:string)
            n119 = flat-sequence {
              tunnel: [w251] -> w234
              tunnel: w235 -> [w251]
              frame #0 {
                n120 = Get Date/Time In Seconds() -> (seconds since 1Jan1904=w252:timestamp)
                n121 = To Double Precision Float(number=w252) -> (double precision float=→"Tiempo":dbl)
                n122 = local write "Developer commad"("" ("Developer commad")) -> ()
                n123 = local write "Adquirir"(FALSE ("Adquirir")) -> ()
              }
            }
          }
          frame "Adquisición" {
            n124 = local read "Watchdog config"() -> (w326:T1)
            n125 = flat-sequence {
              tunnel: w315 -> [w355]
              tunnel: w314 -> [w354]
              tunnel: [w355] -> w313
              tunnel: [w354] -> w312
              frame #0 {
                n126 = local read "Report"() -> (w351:string)
                n127 = call "Reporting_datetime.vi"() -> ("String"=w350:string)  [unwired: 11 in]
                n128 = Concatenate Strings(w350, "\nSTATUS: ACQUISITION\nTrain is passing\n\n", w351) -> (w353:string)
                n129 = local write "Report"(w353) -> ()
              }
            }
            n130 = call <vilib>:"Watchdog Configure.vi"("error in (no error)"=w325, "expiration actions"=w326, "timeout (1 sec)"=200.0) -> ("error out"=w323:errorcluster, "watchdogID"=w324:u64)  [unwired: 1 in, 2 out]
            n131 = flat-sequence {
              tunnel: w312 -> [w389]
              tunnel: w313 -> [w390]
              tunnel: [w388] -> w340
              tunnel: [w387] -> w339
              tunnel: [w386] -> w338
              tunnel: [w385] -> w337
              tunnel: [w384] -> w336
              tunnel: [w383] -> w335
              tunnel: [w373] -> w328
              tunnel: w324 -> [w372]
              tunnel: w323 -> [w371]
              tunnel: [w372] -> w322
              tunnel: [w371] -> w321
              tunnel: [w405] -> w349
              tunnel: [w422] -> w348
              tunnel: [w421] -> w347
              tunnel: [w420] -> w346
              tunnel: [w413] -> w345
              tunnel: w340 -> [w419]
              tunnel: w339 -> [w418]
              tunnel: w338 -> [w417]
              tunnel: w337 -> [w416]
              tunnel: w336 -> [w415]
              tunnel: w335 -> [w414]
              tunnel: w328 -> [w411]
              tunnel: [w410] -> w327
              tunnel: w322 -> [w409]
              tunnel: w321 -> [w408]
              tunnel: [w406] -> w320
              tunnel: w349 -> [w588]
              tunnel: w348 -> [w585]
              tunnel: w347 -> [w584]
              tunnel: w346 -> [w601]
              tunnel: [w622] -> w332
              tunnel: w345 -> [w624]
              tunnel: [w616] -> w342
              tunnel: [w617] -> w344
              tunnel: [w618] -> w343
              tunnel: w327 -> [w597]
              tunnel: w320 -> [w589]
              tunnel: [w589] -> w318
              tunnel: [w588] -> w317
              frame #0 {
                n132 = local read "Offset_rueda WS 1"() -> (w366:fxp<+/-,24,-4>)
                n133 = local read "Offset_rueda WS 2"() -> (w367:fxp<+/-,24,-4>)
                n134 = local read "Frecuencia de muestreo (Hz)"() -> (w381:dbl)
                n135 = local read "Escaneos de la FIFO por canal"() -> (w370:u32)
                n136 = local read "Canal cero WS1?"() -> (w375:bool)
                n137 = local read "Count(mSec)"() -> (w374:u32)
                n138 = local read "Frecuencia de muestreo y módulo CRIO"() -> (w377:T2)
                n139 = local read "Canal cero WS2"() -> (w365:bool)
                n140 = local read "Digital?"() -> (w376:bool)
                n141 = Get Date/Time In Seconds() -> (seconds since 1Jan1904=→"Inicio pasada":timestamp)
                n142 = local read "Nº de acelerómetros"() -> (w363:i32)
                n143 = local read "Nº inductivos"() -> (w364:i32)
                n144 = xnode "Read/Write Control"("FPGA VI Reference In"=w390, "error in"=w389, "Data Rate"=w377, "Digital?"=w376, "Canal cero WS1?"=w375, "Count(mSec)"=w374, "Offset_WS1"=w366, "Offset_WS2"=w367, "Canal cero WS2?"=w365) -> ("FPGA VI Reference Out"=w380:refnum<k20>, "error out"=w379:errorcluster)
                n145 = local read "RFID LR6 on?"() -> (w368:bool)
                n146 = Add(x=w364, y=w363) -> (x+y=w369:i32)
                n147 = case shown="True" w368 {
                  tunnel: [errorcluster {"status"=FALSE, "code"=0, "source"=""} ("error out") w395] -> w373
                  frame False {
                  }
                  frame True {
                    n148 = local read "RFID_LR6_Error"() -> (w396:errorcluster)
                    n149 = call "LH6HD.vi"("error in (no error)"=w396, "Action"=enum16{"Init", "Start", "Read", "Stop", "Exit"}."Start") -> ("error out"=w395:errorcluster)  [unwired: 8 in, 1 out]
                  }
                }
                n150 = call "DMACalc.vi"("Number of Channels"=w369, "Number of Samples"=w370, "Rate (Hz)"=w381) -> ("Block Size"=w385:u32, "Time to Acquire Block (ms)"=w386:i32, "Host Buffer Size"=w391:u32)  [unwired: 6 in]
                n151 = call "Pathhorafech(SubVI)_varios.vi"("Folder path"=path "c:/Trenes", "Nº de acelerómetros"=w363, "Nº inductivos"=w364) -> ("Acel_Paths"=w359:path[])  [unwired: 1 in, 1 out]
                "Nombre de archivo" <- w359
                n152 = Index Array(array=w359) -> (element=w358:path)  [unwired: 1 in]
                n153 = for {
                  tunnel: w359 -> [w400] mode=indexing
                  tunnel: [w399] -> w384 mode=indexing
                  tunnel: [w398] -> w383
                  n154 = Open/Create/Replace File(file path (use dialog)=w400, operation (0:open)=T4."replace or create", access (0:read/write)=enum16{"read/write", "read-only", "write-only"}."read/write", disable buffering (F)=TRUE) -> (refnum out=w399:refnum<file>, error out=w398:errorcluster)  [unwired: 1 in, 2 out]
                }
                n155 = xnode "Invoke Method"("FPGA VI Reference In"=w380, "error in"=w379, "Requested Depth"=w391) -> ("FPGA VI Reference Out"=w393:refnum<k20>, "error out"=w392:errorcluster)  [unwired: 1 out]
                n156 = local read "Report"() -> (w362:string)
                n157 = Path To String(path=w358) -> (string=w356:string)
                n158 = Concatenate Strings("\nFile created: ", w356, "\n", w362) -> (w361:string)
                n159 = xnode "Invoke Method"("FPGA VI Reference In"=w393, "error in"=w392) -> ("FPGA VI Reference Out"=w388:refnum<k20>, "error out"=w387:errorcluster)
                n160 = local write "Report"(w361) -> ()
              }
              frame #1 {
                n161 = while "Data Acquisition" {
                  tunnel: w419 -> [w473]
                  shift-right: [w497] -> _
                  shift-left: u32 0 ("t") -> [w493]
                  tunnel: w417 -> [w498]
                  tunnel: w416 -> [w496]
                  shift-right: [w499] -> w421
                  shift-left: w418 -> [w490]
                  tunnel: [w494] -> w422
                  tunnel: w415 -> [w477]
                  tunnel: [w478] -> w420
                  shift-right: [w476] -> w413
                  shift-left: w414 -> [w486]
                  stop <- w495 stop-if-true
                  # "Detector de presencia"
                  # "Mide el tiempo de paso del tren y con ello se puede calcular\nla velocidad la unidad"
                  n162 = xnode "Invoke Method"("FPGA VI Reference In"=w473, "error in"=w490, "Number of Elements"=w493, "Timeout (ms)"=0) -> ("FPGA VI Reference Out"=w470:refnum<k20>, "error out"=w475:errorcluster, "Data"=w489:fxp<+/-,24,4>[], "Elements Remaining"=w491:u32)
                  n163 = case "Data Ready" shown="Default" w493 {
                    tunnel: w498 -> [w521 _]
                    tunnel: [w520 u32 0 ("t")] -> w497
                    tunnel: w496 -> [w522 _]
                    tunnel: w491 -> [w519 _]
                    tunnel: w489 -> [_ w544]
                    tunnel: w486 -> [w518 w543]
                    tunnel: [w518 w545] -> w476
                    tunnel: w477 -> [w517 w542]
                    tunnel: [w517 w541] -> w478
                    frame 0 {
                      # "En este caso se compara los elementos que quedan\nen la FIFO del controlador con el tamaño dell bloque\nque aparece en el panel frontal. Si el número de \nelementos en la FIFO es mayor o igual que el tamaño\n del bloque se pasa al siguiente caso y se guardan \nlos datos en un archivo. El reloj que aparece es una\nespera para no consumir recursos."
                      n164 = Greater Or Equal?(x=w519, y=w522) -> (x >= y?=w523:bool)
                      n165 = case shown="False" w523 {
                        tunnel: [u32 0 ("Block Size") w527] -> w520
                        tunnel: [w526 0 ("t")] -> w524
                        tunnel: w521 -> [w526 _]
                        tunnel: w522 -> [_ w527]
                        frame False {
                        }
                        frame True {
                        }
                      }
                      n166 = call "WaitMinTimeBetweenCall.vi"("Minimum ms between calls"=w524) -> ()  [unwired: 2 in]
                    }
                    frame Default {
                      n167 = To Single Precision Float(number=w544) -> (single precision float=w531:sgl[])
                      n168 = Decimate 1D Array(w531) -> (w537:sgl[], w540:sgl[], w539:sgl[], w538:sgl[], w536:sgl[], w535:sgl[], w534:sgl[], w533:sgl[], w532:sgl[], w529:sgl[])
                      n169 = Build Array(w537, w540, w539, w538, w536, w535, w534, w533, w532, w529) -> (w530:sgl[][])
                      n170 = for {
                        tunnel: T5."little-endian" ("byte order (0:big-endian, network order)") -> [w554]
                        shift-right: [w548] -> w545
                        shift-left: w543 -> [w549]
                        tunnel: w530 -> [w552] mode=indexing
                        tunnel: w542 -> [w551] mode=indexing
                        tunnel: [w550] -> w541 mode=indexing
                        n171 = Write to Binary File(file (use dialog)=w551, data=w552, error in=w549, 5:FALSE ("prepend array or string size? (T)"), 9:w554) -> (refnum out=w550:refnum<file>, error out=w548:errorcluster)  [unwired: 2 out]
                      }
                    }
                  }
                  n172 = xnode "Read/Write Control"("FPGA VI Reference In"=w470, "error in"=w475) -> ("FPGA VI Reference Out"=w488:refnum<k20>, "error out"=w487:errorcluster, "Parar"=w466:bool, "Nº Ruedas 1"=→"Nº Ruedas 1":i32, "NºRuedas 2"=→"NºRuedas 2":i32)
                  "Parar" <- w466
                  n173 = case shown="True" w466 {
                    tunnel: [w504 w512] -> w467
                    tunnel: [w505 0.0] -> w481
                    frame False {
                      n174 = local read "Inicio pasada"() -> (w508:timestamp)
                      n175 = Get Date/Time In Seconds() -> (seconds since 1Jan1904=w507:timestamp)
                      n176 = local read "Tiempo de adquisicion"() -> (w500:dbl)
                      n177 = To Double Precision Float(number=w507) -> (double precision float=w506:dbl)
                      n178 = To Double Precision Float(number=w508) -> (double precision float=w509:dbl)
                      n179 = Subtract(x=w506, y=w509) -> (x-y=w505:dbl)
                      "Tiempo de paso (s)" <- w505
                      n180 = local write "Tiempo"(w506) -> ()
                      n181 = local read "Boton Adquirir?"() -> (w501:bool)
                      n182 = Greater?(x=w505, y=w500) -> (0:w503:bool)
                      n183 = Select(t=w503, s=w501, f=FALSE) -> (s? t:f=w504:bool)
                    }
                    frame True {
                      n184 = local read "Tiempo"() -> (w516:dbl)
                      n185 = local read "Tiempo extra al detector de paso (s)"() -> (w511:dbl)
                      n186 = Get Date/Time In Seconds() -> (seconds since 1Jan1904=w513:timestamp)
                      n187 = To Double Precision Float(number=w513) -> (double precision float=w514:dbl)
                      n188 = Subtract(x=w514, y=w516) -> (x-y=w515:dbl)
                      n189 = Greater?(x=w515, y=w511) -> (0:w512:bool)
                    }
                  }
                  "Fin" <- w467
                  n190 = local read "Timeout ruedas"() -> (w465:dbl)
                  n191 = xnode ("CheckLate")("FPGA VI Reference In"=w488, "error in"=w487) -> ("FPGA VI Reference Out"=w472:refnum<k20>, "error out"=w483:errorcluster, "Buffer Underflow"=→"Buffer Underflow":bool, "Buffer Overflow"=w474:bool)
                  "Buffer Overflow" <- w474
                  n192 = Greater?(x=w481, y=w465) -> (0:w479:bool)
                  "Timeout ruedas" <- w479
                  n193 = call "ErrorOverFlow.vi"("Buffer Overflow"=w474) -> ("error out"=w482:errorcluster)
                  n194 = Merge Errors(w483, w482) -> (w471:errorcluster)
                  n195 = Unbundle By Name(w476) -> ("status"=w480:bool)
                  n196 = Unbundle By Name(w471) -> ("status"=w485:bool)
                  n197 = Compound Arithmetic op=OR(w485, w467, w479, w480) -> (w495:bool)
                  "result" <- w495
                  n198 = case "Flush" shown="True" w495 {
                    tunnel: [w555 w560] -> w499
                    tunnel: [w556 w559] -> w494
                    tunnel: w472 -> [w556 w558]
                    tunnel: w471 -> [w555 w557]
                    frame False {
                    }
                    frame True {
                      n199 = xnode "Invoke Method"("FPGA VI Reference In"=w558, "error in"=w557) -> ("FPGA VI Reference Out"=w559:refnum<k20>, "error out"=w560:errorcluster)
                    }
                  }
                  "Block Size" <- w496
                  "Time to Acquire Block (ms)" <- w498
                }
                n200 = call <vilib>:"Watchdog Whack.vi"("error in (no error)"=w408, "reset watchdog after expire? (F)"=TRUE, "watchdogID in"=w409) -> ("error out"=w405:errorcluster, "watchdogID out"=w406:u64)  [unwired: 2 in, 1 out]
                n201 = local read "RFID LR6 on?"() -> (w404:bool)
                n202 = case shown="True" w404 {
                  tunnel: w411 -> [w423 w429]
                  tunnel: [w423 w428] -> w410
                  frame False {
                  }
                  frame True {
                    n203 = while {
                      shift-right: [w436] -> w428
                      shift-left: w429 -> [w437]
                      shift-right: [w435] -> w426
                      shift-left: string[] [] -> [w434]
                      shift-right: [w430] -> w424
                      shift-left: i32[] [] -> [w431]
                      i -> [w432]
                      stop <- w433 stop-if-true
                      n204 = case shown="No Error" w437 {
                        selector: w437 -> [w448 _]
                        tunnel: [w447 w463] -> w436
                        tunnel: [w443 string[] []] -> w435
                        tunnel: w434 -> [w442 _]
                        tunnel: w432 -> [w441 _]
                        tunnel: w431 -> [w440 _]
                        tunnel: [w439 i32[] []] -> w430
                        frame No Error {
                          n205 = call "LH6HD.vi"("error in (no error)"=w448, "Action"=enum16{"Init", "Start", "Read", "Stop", "Exit"}."Read") -> ("error out"=w447:errorcluster, "Tag"=w444:string)  [unwired: 8 in]
                          n206 = Not Equal?(x="", y=w444) -> (x != y?=w445:bool)
                          n207 = case shown="False" w445 {
                            tunnel: w444 -> [_ w457]
                            tunnel: [w451 w456] -> w443
                            tunnel: w442 -> [w451 w455]
                            tunnel: w441 -> [_ w452]
                            tunnel: w440 -> [w450 w454]
                            tunnel: [w450 w453] -> w439
                            frame False {
                            }
                            frame True {
                              n208 = Build Array (concatenate)(w455, w457) -> (w456:string[])
                              n209 = Build Array (concatenate)(w454, w452) -> (w453:i32[])
                            }
                          }
                        }
                        frame Error {
                          n210 = local read "LR6 IP address"() -> (w460:string)
                          n211 = local read "DeviceAddress"() -> (w458:u8)
                          n212 = local read "Port LR6"() -> (w461:u16)
                          n213 = call "LH6HD.vi"("DeviceAddress"=w458, "Reader Port"=w461, "IP Address"=w460, "Action"=enum16{"Init", "Start", "Read", "Stop", "Exit"}."Init") -> ("error out"=w463:errorcluster)  [unwired: 6 in, 1 out]
                        }
                      }
                      n214 = Wait Until Next ms Multiple(millisecond multiple=u32 500) -> ()  [unwired: 1 out]
                      n215 = local read "result"() -> (w433:bool)
                      "it-LR6" <- w432
                    }
                    "TAGs LR6" <- w426
                    "it-read-LR6" <- w424
                  }
                }
              }
              frame #2 {
                # "Antes se miraba timeout ruedas"
                # "ORGANIZAR\nTAGS AQUÍ"
                n216 = local read "RFID LR6 on?"() -> (w586:bool)
                n217 = local read "RFID NEM on?"() -> (w587:bool)
                n218 = Array Size(array=w601) -> (size(s)=w599:i32)
                n219 = local read "AURA wheel test"() -> (w568:bool)
                n220 = Decrement(x=w599) -> (x-1=w600:i32)
                n221 = case shown="True" w586 {
                  tunnel: w597 -> [w644 w650]
                  tunnel: [w644 w645] -> w596
                  frame False {
                  }
                  frame True {
                    n222 = call "LH6HD.vi"("error in (no error)"=w650, "Action"=enum16{"Init", "Start", "Read", "Stop", "Exit"}."Stop") -> ("error out"=w645:errorcluster)  [unwired: 8 in, 1 out]
                    n223 = call "Reporting_error.vi"("error out 2"=w645, "Concept"="Active RFID") -> ("Reporting"=w647:string)  [unwired: 1 in]
                    n224 = local read "Report"() -> (w648:string)
                    n225 = Concatenate Strings(w647, w648) -> (w646:string)
                    n226 = local write "Report"(w646) -> ()
                  }
                }
                n227 = case shown="True" w587 {
                  tunnel: [string[] [] ("TagArray") w657] -> w562
                  tunnel: [cluster{"TagCode":string, "FirstSeemUs":u64}[] [] ("TagData out") w656] -> w566
                  frame False {
                  }
                  frame True {
                    n228 = call "IF2_TagBuffer.vi"("Action"=enum16{"Init", "WriteTagData", "ReadTagData"}."ReadTagData") -> ("error out"=w655:errorcluster, "TagData out"=w656:cluster{"TagCode":string, "FirstSeemUs":u64}[])  [unwired: 9 in]
                    n229 = local read "connection ID"() -> (w654:refnum<k5>)
                    n230 = call "RFID_TAGS_Sort.vi"("TagData in"=w656) -> ("TagString"=w658:string, "TagArray"=w657:string[])  [unwired: 9 in]
                    n231 = call "IF2_Clear_buffer.vi"("error in (no error)"=w655, "TCP Network Connection in"=w654) -> ()  [unwired: 8 in, 2 out]
                    n232 = call "Reporting_error.vi"("error out 2"=w655, "Concept explanation"=w658, "Concept"="Passive RFID") -> ("Reporting"=w661:string)
                    n233 = local read "Report"() -> (w662:string)
                    n234 = Concatenate Strings(w661, w662) -> (w660:string)
                    n235 = local write "Report"(w660) -> ()
                  }
                }
                "TAGs HEX" <- w562
                n236 = Index Array(array=w601, index=w600) -> (element=w609:refnum<file>)
                n237 = local write "result"(FALSE ("result")) -> ()
                n238 = xnode "Read/Write Control"("FPGA VI Reference In"=w585, "error in"=w584) -> ("FPGA VI Reference Out"=w621:refnum<k20>, "error out"=w582:errorcluster, "Chassis Temperature"=w629:i16)
                n239 = local read "TAGs LR6"() -> (w570:string[])
                n240 = Select(t=string[] ["A0000000000000000TESTNEM7", "A0000000000000000TESTNEM8"], s=w568, f=w570) -> (s? t:f=w567:string[])
                n241 = Divide(x=w629, y=4.0) -> (x/y=w579:dbl)
                "Temperatura (ºC)" <- w579
                n242 = local read "Tiempo de paso (s)"() -> (w620:dbl)
                n243 = for {
                  tunnel: w567 -> [w666] mode=indexing
                  tunnel: [w664] -> w590 mode=indexing
                  n244 = Search and Replace String(input string=w666, search string="00") -> (result string=w664:string)  [unwired: 6 in, 3 out]
                }
                n245 = local write "RFID_LR6_Error"(w596) -> ()
                n246 = Index Array(array=w562) -> (element=w595:string)  [unwired: 1 in]
                n247 = local read "Nº Ruedas 1"() -> (w577:i32)
                n248 = local read "NºRuedas 2"() -> (w580:i32)
                n249 = Not Equal?(x=w595, y="" ("delimiter (\\t)")) -> (x != y?=w593:bool)
                "Plataformas?" <- w593
                n250 = Multiply(x=w620, y=1000.0) -> (x*y=w578:dbl)
                n251 = case shown="True" w593 {
                  tunnel: w590 -> [w667 w673]
                  tunnel: [w667 w672] -> _
                  tunnel: w562 -> [_ _]
                  tunnel: w566 -> [_ w668]
                  frame False {
                  }
                  frame True {
                    n252 = local read "Tiempo de paso (s)"() -> (w670:dbl)
                    n253 = local read "Tabla_flota"() -> (w669:string[][])
                    n254 = local read "Inicio pasada"() -> (w671:timestamp)
                    n255 = call "Union_TAGs_RFIDs.vi"("TAGs LR6"=w673) -> ()  [unwired: 1 in, 1 out]
                    n256 = call "TagNormalizaction.vi"("Inicio pasada"=w671, "Tiempo de paso (s)"=w670, "TagData in"=w668, "Tabla_flota"=w669) -> ("Normalized Tags"=w672:string[])  [unwired: 7 in]
                  }
                }
                n257 = Build Array(w579, w578, w577, w580) -> (w581:dbl[])
                n258 = Build Array(w579, w578, w577) -> (w576:dbl[])
                n259 = local read "Leer config RFID NEM"() -> (w564:bool)
                n260 = Array Size(array=w562) -> (size(s)=w563:i32)
                n261 = for {
                  N: w563 -> [_]
                  shift-right: [w631] -> w561
                  shift-left: w562 -> [w633]
                  n262 = Search 1D Array(1D array=w633, element="") -> (index of element=w630:i32)  [unwired: 1 in]
                  n263 = Delete From Array(array=w633, index=w630) -> (array with subset deleted=w631:string[])  [unwired: 1 in, 1 out]
                }
                "TAGs" <- w561
                n264 = local read "Direccion 0?"() -> (w575:bool)
                n265 = case shown="True" w564 {
                  tunnel: w562 -> [_ w634]
                  frame False {
                  }
                  frame True {
                    n266 = Format Date/Time String(time format string (%c)="%Y-%m-%d-%H-%M-%S") -> (date/time string=w641:string)  [unwired: 2 in]
                    n267 = Concatenate Strings("/c/RFID/", w641, ".csv" ("element")) -> (w639:string)
                    n268 = String To Path(string=w639) -> (path=w635:path)
                    n269 = call-poly <vilib>:"Write Delimited Spreadsheet.vi"("file path (dialog if empty)"=w635, "1D data"=w634, "append to file? (F)"=TRUE, "transpose? (F)"=TRUE, "delimiter (\\t)"=";" ("delimiter (\\t)")) -> ()  [unwired: 9 in, 2 out]
                  }
                }
                n270 = local read "Nombre de archivo"() -> (w608:path[])
                n271 = Bundle("error out"=w582, w581, "TagArray"=w561, "Direccion 0?"=w575) -> (w574:T10)  [unwired: 1 in]
                n272 = for {
                  shift-right: [w679] -> w614
                  shift-left: string[] [] -> [w678]
                  tunnel: w561 -> [w677] mode=indexing
                  n273 = Insert Into Array(array=w678, new element=w677) -> (w679:string[])  [unwired: 1 in]
                }
                n274 = xnode "Read/Write Control"("FPGA VI Reference In"=w621, "error in"=w582, "Stop"=TRUE ("stop")) -> ("FPGA VI Reference Out"=w611:refnum<k20>, "error out"=w610:errorcluster)
                n275 = call "Reporting_acqu.vi"("output cluster"=w574, "address repoting"=path "C:/Reporting/Reporting_adqu.txt" ("file (use dialog)")) -> ("Reporting"=w571:string)  [unwired: 1 in]
                n276 = Delete From Array(array=w608) -> (deleted portion=w607:path)  [unwired: 2 in, 1 out]
                n277 = local read "Report"() -> (w572:string)
                n278 = To Single Precision Float(number=w576) -> (single precision float=w627:sgl[])
                n279 = Path To String(path=w607) -> (string=w613:string)
                n280 = Concatenate Strings(w571, w572) -> (w573:string)
                n281 = Write to Binary File(file (use dialog)=w609, data=w627, error in=w624, 5:FALSE ("prepend array or string size? (T)"), 9:T5."little-endian" ("byte order (0:big-endian, network order)")) -> (error out=w606:errorcluster)  [unwired: 3 out]
                n282 = xnode "Invoke Method"("FPGA VI Reference In"=w611, "error in"=w610) -> ("FPGA VI Reference Out"=w618:refnum<k20>, "error out"=w617:errorcluster)
                n283 = local write "Report"(w573) -> ()
                n284 = Build Array (concatenate)(w613, w614) -> (w591:string[])
                n285 = local read "TAGS leidos"() -> (w602:path)
                n286 = for {
                  shift-right: [w676] -> w616
                  shift-left: w606 -> [w675]
                  tunnel: w601 -> [w674] mode=indexing
                  n287 = Close File(refnum=w674, error in=w675) -> (error out=w676:errorcluster)  [unwired: 1 out]
                }
                n288 = call-poly <vilib>:"Write Delimited Spreadsheet.vi"("file path (dialog if empty)"=w602, "1D data"=w591, "append to file? (F)"=TRUE ("transpose? (no:F)"), "transpose? (F)"=TRUE ("append to file? (new file:F)"), "delimiter (\\t)"=";" ("delimiter (\\t)")) -> ()  [unwired: 9 in, 2 out]
                n289 = Select(t="TEST", s=FALSE, f="Procesado") -> (s? t:f=w622:string)
              }
            }
            n290 = call <vilib>:"Watchdog Clear.vi"("error in (no error)"=w317, "watchdogID in"=w318) -> ("error out"=w319:errorcluster)  [unwired: 5 in]
            n291 = Unbundle By Name(w344) -> ("status"=w333:bool)
            n292 = Unbundle By Name(w342) -> ("status"=w334:bool)
            n293 = Merge Errors(w342, w319) -> (w341:errorcluster)
            n294 = Compound Arithmetic op=OR(w333, w334) -> (w331:bool)
            n295 = Select(t="TEST", s=w331, f=w332) -> (s? t:f=w329:string)
          }
          frame "Procesado" {
            n296 = local read "Watchdog config"() -> (w691:T1)
            n297 = flat-sequence {
              tunnel: w685 -> [w704]
              tunnel: [w704] -> w684
              tunnel: w683 -> [w700]
              tunnel: [w700] -> w682
              frame #0 {
                n298 = local read "Report"() -> (w701:string)
                n299 = call "Reporting_datetime.vi"() -> ("String"=w699:string)  [unwired: 11 in]
                n300 = Concatenate Strings(w699, "\nSTATUS: PROCESSING\nProcessing the measurement\n\n", w701) -> (w703:string)
                n301 = local write "Report"(w703) -> ()
              }
            }
            n302 = call <vilib>:"Watchdog Configure.vi"("error in (no error)"=w694, "expiration actions"=w691, "timeout (1 sec)"=300.0) -> ("error out"=w693:errorcluster, "watchdogID"=w690:u64)  [unwired: 1 in, 2 out]
            n303 = flat-sequence {
              tunnel: w693 -> [w711]
              tunnel: w690 -> [w707]
              tunnel: [w706] -> w689
              tunnel: [w705] -> w688
              tunnel: [w962] -> w687
              tunnel: w689 -> [w962]
              tunnel: [w961] -> w686
              tunnel: w688 -> [w961]
              frame #0 {
                n304 = flat-sequence {
                  tunnel: [w785] -> w713
                  tunnel: [w715] -> w712
                  tunnel: w711 -> [w756]
                  tunnel: [w739] -> w708
                  tunnel: [w773] -> w710
                  tunnel: [w730] -> w709
                  tunnel: w707 -> [w757]
                  tunnel: [w754] -> w706
                  tunnel: [w753] -> w705
                  frame #0 {
                    n305 = local read "AURA wheel test"() -> (w728:bool)
                    n306 = case shown="False" w728 {
                      tunnel: [w788 w789] -> w727
                      tunnel: [w787 path[] [path "c:/Trenes_prueba/A_0_TEST.bin", path "c:/Trenes_prueba/A_1_TEST.bin", path "c:/Trenes_prueba/A_2_TEST.bin", path "c:/Trenes_prueba/A_3_TEST.bin", path "c:/Trenes_prueba/A_4_TEST.bin", path "c:/Trenes_prueba/A_5_TEST.bin", path "c:/Trenes_prueba/A_6_TEST.bin", path "c:/Trenes_prueba/A_7_TEST.bin", path "c:/Trenes_prueba/I_0_TEST.bin", path "c:/Trenes_prueba/I_1_TEST.bin"]] -> w726
                      frame False {
                        n307 = local read "Nombre de archivo"() -> (w787:path[])
                        n308 = local read "TAGs"() -> (w788:string[])
                      }
                      frame True {
                        w789 = string[] ["A0000000000000000TESTNEM7", "A0000000000000000TESTNEM8"]
                        n309 = local write "TAGs LR6"(w789) -> ()
                      }
                    }
                    n310 = local read "Tabla_flota"() -> (w772:string[][])
                    n311 = call <vilib>:"Watchdog Whack.vi"("error in (no error)"=w756, "reset watchdog after expire? (F)"=TRUE, "watchdogID in"=w757) -> ("error out"=w753:errorcluster, "watchdogID out"=w754:u64)  [unwired: 2 in, 1 out]
                    n312 = local read "Puntos medios de las ventanas"() -> (w718:dbl[][])
                    n313 = call "Series_ejes_flota.vi"("Tabla_flota"=w772, "Tags"=w727) -> ("Nº Ejes"=w719:i32[], "Series del convoy"=w720:string[])  [unwired: 2 in, 1 out]
                    "Nº Ejes" <- w719
                    n314 = Array Size(array=w726) -> (size(s)=w779:i32)
                    n315 = Add Array Elements(numeric array=w719) -> (sum=w738:i32)
                    "Ejes_convoy" <- w738
                    n316 = local read "Series_flota"() -> (w717:string[])
                    n317 = Subtract(x=w779, y=2 ("length")) -> (x-y=w781:i32)
                    n318 = Array Size(array=w720) -> (size(s)=→"Nº UTs":i32)
                    n319 = local read "Radios ruedas"() -> (w716:dbl[])
                    n320 = Delete From Array(array=w726, length=2, index=w781) -> (deleted portion=w758:path[], array with subset deleted=w773:path[])
                    n321 = Index Array(array=w758) -> (element #2=w752:path)  [unwired: 2 in, 1 out]
                    n322 = call "Distancias_ejes_convoy_baja_velocidad.vi"("Radios ruedas"=w716, "Series_flota1"=w720, "Ejes_UT"=w719, "Puntos medios de las ventanas"=w718, "Series_flota"=w717) -> ("Radios_por_ejes"=→"Radios_por_ejes":dbl[], "Distancias_entre_ejes_convoy"=w715:dbl[])  [unwired: 1 in]
                    n323 = Read from Binary File(5:sgl 0.0, 9:T5."little-endian" ("byte order (0:big-endian, network order)"), 10:-1 ("count (1)"), 11:w752) -> (0:w777:errorcluster, 2:w760:sgl[], 3:w778:refnum<file>)  [unwired: 1 in, 2 out]
                    n324 = local read "Frecuencia de muestreo (Hz)"() -> (w743:dbl)
                    n325 = local read "Offset_rueda WS 2"() -> (w744:fxp<+/-,24,-4>)
                    n326 = local read "it-LR6"() -> (w763:i32)
                    n327 = local read "it-read-LR6"() -> (w764:i32[])
                    n328 = local read "TAGs LR6"() -> (w765:string[])
                    n329 = local read "Plataformas?"() -> (w762:bool)
                    n330 = local read "TAGs"() -> (w766:string[])
                    n331 = Close File(refnum=w778, error in=w777) -> (error out=w722:errorcluster)  [unwired: 1 out]
                    n332 = Array Size(array=w760) -> (size(s)=w771:i32)
                    n333 = Subtract(x=w771, y=3 ("length")) -> (x-y=w769:i32)
                    n334 = Delete From Array(array=w760, length=3, index=w769) -> (array with subset deleted=w750:sgl[])  [unwired: 1 out]
                    n335 = call "TAGs_AURAwheel_TAGM_NEM.vi"("Nº Ejes"=w719, "TAGs"=w766, "Ejes_convoy"=w738, "it-LR6"=w763, "TAGs LR6"=w765, "it-read-LR6"=w764, "Plataformas?"=w762) -> ("TAGS_AURA"=→"TAGs_AURAwheel":string[][])  [unwired: 1 in]
                    n336 = call "Analogico_digital.vi"("Array"=w750, "Offset WS"=w744, "Frecuencia muestreo"=w743) -> ("array w/ subset deleted"=w745:sgl[], "Tiempo\npaso"=w742:dbl)  [unwired: 6 in]
                    n337 = call "Puntos medio de pulso.vi"("DI Inductivo"=w745) -> ("Puntos"=w785:sgl[], "Número de ejes"=w732:i32)  [unwired: 1 in]
                    "Número de ejes detectados" <- w732
                    n338 = disable-structure shown="Enabled" {
                      disable-tunnel: w750 -> [w797 w800]
                      disable-tunnel: [FALSE ("element") TRUE ("element")] -> w747
                      disable-tunnel: [w791 w799] -> w746
                      frame Disabled {
                        n339 = Equal?(x=w797, y=0.0) -> (x = y?=w794:bool[])
                        n340 = Equal?(x=w797, y=1.0) -> (x = y?=w795:bool[])
                        n341 = Or(x=w794, y=w795) -> (x .or. y?=w791:bool[])
                      }
                      frame Enabled {
                        n342 = Greater?(x=w800, y=0.1) -> (0:w799:bool[])
                      }
                    }
                    n343 = Decrement(x=w732) -> (x-1=w784:i32)
                    n344 = call "Reporting_error.vi"("error out 2"=w722, "Concept"="Measurement reading") -> ("Reporting"=w724:string)  [unwired: 1 in]
                    n345 = Get Volume Info(11:path "c:/" ("path")) -> (1:w733:i64)  [unwired: 1 in, 5 out]
                    "Disco Duro Disponible (bytes)" <- w733
                    n346 = local read "Report"() -> (w725:string)
                    n347 = call "Calculo_Velocidad.vi"("Tiempo de paso (s)"=w742, "Ejes"=w784, "Puntos iniciales de las ventanas"=w715) -> ("V (m/s)"=→"V (m/s)":dbl, "Longitud de la unidad"=→"Longitud de la unidad":dbl)
                    n348 = Concatenate Strings(w724, w725) -> (w723:string)
                    n349 = Equal?(x=w738, y=w732) -> (x = y?=w730:bool)
                    n350 = Not Equal?(x=w732, y=0) -> (x != y?=w729:bool)
                    n351 = Search 1D Array(1D array=w746, element=w747) -> (index of element=w748:i32)  [unwired: 1 in]
                    n352 = local write "Report"(w723) -> ()
                    n353 = Build Array(w738, w732, w733) -> (w737:i64[])
                    n354 = Equal?(x=w748, y=-1) -> (x = y?=w751:bool)
                    n355 = Compound Arithmetic op=AND(w730, w729, w751) -> (w739:bool)
                    "Archivo\nvalido?" <- w739
                    n356 = Bundle(w737, w739) -> (w735:cluster{i64[], bool})  [unwired: 1 in]
                    n357 = call "Reporting_proc.vi"("output cluster 2"=w735, "address repoting"=path "C:/Reporting/Reporting_proc.txt" ("file (use dialog)")) -> ("Reporting"=w734:string)  [unwired: 1 in]
                    n358 = local read "Report"() -> (w740:string)
                    n359 = Concatenate Strings(w734, w740) -> (w741:string)
                    n360 = local write "Report"(w741) -> ()
                  }
                }
                n361 = case shown="True" w708 {
                  tunnel: w713 -> [_ w838]
                  tunnel: w712 -> [_ w836]
                  tunnel: w710 -> [_ w837]
                  tunnel: w709 -> [w802 _]
                  frame False {
                    n362 = local read "Nombre de archivo"() -> (w803:path[])
                    n363 = for {
                      tunnel: w803 -> [w805] mode=indexing
                      tunnel: w802 -> [w804]
                      n364 = flat-sequence {
                        tunnel: w805 -> [w815]
                        tunnel: [w815] -> w808
                        tunnel: [w814] -> w807
                        tunnel: w804 -> [w813]
                        tunnel: w808 -> [w822]
                        tunnel: [w821] -> w806
                        tunnel: w807 -> [w821]
                        tunnel: w806 -> [w824]
                        frame #0 {
                          w814 = path "c:/Est_Adq.csv" ("file path (use dialog)")
                          n365 = Path To String(path=w815) -> (string=w816:string)
                          n366 = Select(t="Nº Ejes detectados WS diferente a Nº Ejes TAGs" ("delimiter (\\t)"), s=w813, f="La señal del inductivo no es digital" ("delimiter (\\t)")) -> (s? t:f=w810:string)
                          n367 = Build Array(w816, w810) -> (w809:string[])
                          n368 = call-poly <vilib>:"Write Delimited Spreadsheet.vi"("file path (dialog if empty)"=w814, "1D data"=w809, "append to file? (F)"=FALSE ("transpose? (no:F)"), "transpose? (F)"=TRUE ("append to file? (new file:F)"), "delimiter (\\t)"=";" ("delimiter (\\t)")) -> ()  [unwired: 9 in, 2 out]
                        }
                        frame #1 {
                          n369 = local read "Borrar archivos\nadquisicion con error"() -> (w820:bool)
                          n370 = case shown="True" w820 {
                            tunnel: w822 -> [_ w823]
                            frame False {
                            }
                            frame True {
                              n371 = Delete(path (use dialog)=w823) -> ()  [unwired: 1 in, 6 out]
                            }
                          }
                        }
                        frame #2 {
                          n372 = File/Directory Info(path=w824) -> (size=w827:i64)  [unwired: 1 in, 6 out]
                          n373 = Greater?(x=w827, y=i64 1000000) -> (0:w825:bool)
                          n374 = case shown="True" w825 {
                            tunnel: w824 -> [_ w828]
                            frame False {
                            }
                            frame True {
                              n375 = Delete(path (use dialog)=w828) -> ()  [unwired: 4 in, 3 out]
                            }
                          }
                        }
                      }
                    }
                  }
                  frame True {
                    n376 = flat-sequence {
                      tunnel: w838 -> [w936]
                      tunnel: w837 -> [w942]
                      tunnel: w836 -> [w935]
                      tunnel: [w923] -> w835
                      tunnel: [w916] -> w829
                      tunnel: [w915] -> w830
                      tunnel: [w914] -> w831
                      frame #0 {
                        # "SALIDA \n\nMáximos por rueda inductivo"
                        # "8 acelerómetros"
                        # "Velocidad"
                        n377 = local read "Frecuencia de muestreo (Hz)"() -> (w939:dbl)
                        n378 = local read "Distancia de acelerómetros"() -> (w947:dbl[])
                        n379 = local read "Parámetros acelerómetros"() -> (w938:dbl[])
                        n380 = local read "Distancias generales"() -> (w940:dbl[])
                        n381 = local read "Número de ejes detectados"() -> (w943:i32)
                        n382 = local read "dt RMS"() -> (w937:dbl)
                        n383 = local read "Radios_por_ejes"() -> (w934:dbl[])
                        n384 = local read "Direccion 0?"() -> (w945:bool)
                        n385 = Index Array(array=w940, index=1) -> (element=w950:dbl)
                        n386 = local read "freq_cuthigh"() -> (w918:dbl)
                        n387 = local read "freq_cutlow"() -> (w917:dbl)
                        n388 = Select(t=0.0, s=w945, f=w950) -> (s? t:f=w948:dbl)
                        n389 = Subtract(x=w948, y=w947) -> (x-y=w946:dbl[])
                        n390 = Absolute Value(x=w946) -> (abs(x)=w941:dbl[])
                        n391 = call "Procesado_aRMS_BIdirecc_Freq_Energia.vi"("Distancias centrales de las ruedas\n               configuración (m)"=w935, "Puntos"=w936, "dt RMS 2"=w937, "Parámetros acelerómetros"=w938, "Frecuencia de muestreo"=w939, "Distancias generales (m)"=w940, "Radios por ejes"=w934, "high cutoff freq: fh"=w918, "low cutoff freq: fl"=w917, "Ejes Procesados"=w943, "Distancias\nacelerometros"=w941, "Paths_canales_aRMS"=w942) -> ("Max RMS Ruedas"=w933:dbl[][], "Frecuencias de rueda"=w922:dbl[][], "Amplitudes"=w921:dbl[][], "Energía"=w920:dbl[][])  [unwired: 4 in]
                        n392 = Transpose 2D Array(2D array=w933) -> (transposed array=w923:dbl[][])
                        "Max RMS Ruedas" <- w923
                        n393 = Transpose 2D Array(2D array=w921) -> (transposed array=w915:dbl[][])
                        n394 = Transpose 2D Array(2D array=w920) -> (transposed array=w916:dbl[][])
                        n395 = Transpose 2D Array(2D array=w922) -> (transposed array=w914:dbl[][])
                        n396 = call "Reporting_proc_RMS_inycom.vi"("Max RMS Ruedas"=w923) -> ("String"=w929:string)
                        n397 = call "Reporting_proc_energia_inycom.vi"("Datos"=w914) -> ("String"=w932:string)
                        n398 = call "Reporting_proc_energia_inycom.vi"("Datos"=w915) -> ("String"=w931:string)
                        n399 = call "Reporting_proc_energia_inycom.vi"("Datos"=w916) -> ("String"=w930:string)
                        n400 = Concatenate Strings("Max RMS--> " ("string"), w929, "Frequency--> " ("string"), w932, "Amplitude--> " ("string"), w931, "Energy--> " ("string"), w930) -> (w924:string)
                        n401 = local read "Report"() -> (w919:string)
                        n402 = Concatenate Strings(w924, w919) -> (w944:string)
                        n403 = local write "Report"(w944) -> ()
                      }
                    }
                    n404 = local read "TAGs_AURAwheel"() -> (w833:string[][])
                    n405 = local read "Use Aura?"() -> (w834:bool)
                    n406 = local read "Nº Ejes"() -> (w832:i32[])
                    n407 = for {
                      tunnel: w834 -> [w848]
                      tunnel: w833 -> [w847] mode=indexing
                      shift-right: [w846] -> _
                      shift-left: w835 -> [w849]
                      tunnel: w832 -> [w845] mode=indexing
                      shift-right: [w839] -> _
                      shift-left: w831 -> [w844]
                      shift-right: [w840] -> _
                      shift-left: w830 -> [w843]
                      shift-right: [w841] -> _
                      shift-left: w829 -> [w842]
                      # "dev.api.aurawheel.com"
                      n408 = case shown="False" w848 {
                        tunnel: w849 -> [w853 w885]
                        tunnel: w847 -> [_ w866]
                        tunnel: [w853 w884] -> w846
                        tunnel: w845 -> [_ w864]
                        tunnel: w844 -> [w852 w859]
                        tunnel: w843 -> [w851 w858]
                        tunnel: w842 -> [w850 w857]
                        tunnel: [w850 w856] -> w841
                        tunnel: [w851 w855] -> w840
                        tunnel: [w852 w854] -> w839
                        frame False {
                        }
                        frame True {
                          w874 = "\n"
                          w863 = 0 ("index (row)")
                          w890 = cluster{"status":string} {"status"=""}
                          n409 = local read "Parametros AuraWheel"() -> (w913:string[])
                          n410 = Delete From Array(array=w885, length=w864, index (row)=w863) -> (deleted portion=w867:dbl[][], array with subset deleted=w884:dbl[][])  [unwired: 1 in]
                          n411 = Delete From Array(array=w858, length=w864, index (row)=w863) -> (deleted portion=w861:dbl[][], array with subset deleted=w855:dbl[][])  [unwired: 1 in]
                          n412 = Delete From Array(array=w857, length=w864, index (row)=w863) -> (deleted portion=w860:dbl[][], array with subset deleted=w856:dbl[][])  [unwired: 1 in]
                          n413 = Delete From Array(array=w859, length=w864, index (row)=w863) -> (deleted portion=w862:dbl[][], array with subset deleted=w854:dbl[][])  [unwired: 1 in]
                          n414 = Get Date/Time In Seconds() -> (seconds since 1Jan1904=w911:timestamp)
                          n415 = Format Date/Time String(time format string (%c)="%H:%M:%S%3u", seconds (now)=w911) -> (date/time string=w909:string)  [unwired: 1 in]
                          n416 = Scan From String(format string="%d:%d:%f", input string=w909) -> (output 1=w906:i32, output 2=w905:i32, output 3=w903:dbl)  [unwired: 5 in, 3 out]
                          n417 = local read "V (m/s)"() -> (w880:dbl)
                          n418 = local read "Temperatura (ºC)"() -> (w865:dbl)
                          n419 = Get Date/Time In Seconds() -> (seconds since 1Jan1904=w886:timestamp)
                          n420 = Multiply(x=w880, y=3.6) -> (x*y=w870:dbl)
                          n421 = Multiply(x=w903, y=1000.0) -> (x*y=w899:dbl)
                          n422 = Multiply(x=w905, y=60000) -> (x*y=w900:i32)
                          n423 = Multiply(x=3600000, y=w906) -> (x*y=w901:i32)
                          n424 = call "Time_to_ms.vi"("seconds since 1Jan1904"=w886) -> ("Numeric"=w869:dbl)  [unwired: 1 in]
                          n425 = Index Array(array=w913) -> (element #1=w883:string, element #2=w882:string, element #3=w881:string)  [unwired: 3 in]
                          n426 = call "aw_WRDCluster_8acel_baja_velocidad.vi"("TimeStamp"=w869, "p_tp"=w865, "p_sp"=w870, "Array TAGs"=w866, "Energía"=w860, "Amplitudes"=w861, "Frecuencia Ruedas"=w862, "Max RMS Ruedas"=w867) -> ("JSON cluster"=w868:T11)  [unwired: 3 in]
                          n427 = Compound Arithmetic op=ADD(w901, w900, w899) -> (w898:dbl)
                          n428 = To Variant(anything=w868) -> (Variant=w895:variant)
                          n429 = To Unsigned Long Integer(number=w898) -> (unsigned 32bit integer=w897:u32)
                          n430 = call "gjson_Create.vi"("JSON Object in"=w895) -> ("error out"=w893:errorcluster, "JSON String Out"=w894:string)  [unwired: 9 in]
                          n431 = Number To Decimal String(number=w897) -> (decimal integer string=w896:string)  [unwired: 1 in]
                          n432 = To Variant(anything=w890) -> (Variant=w889:variant)
                          n433 = call "aw_SendData.vi"("pwd"=w883, "x-nem-datetime"=w896, "User"=w882, "error in"=w893, "JSON Object"=w894, "URL"=w881) -> ("error out"=w891:errorcluster, "Response JSON"=w892:string, "Response headers"=w875:string)  [unwired: 3 in]
                          "Response headers" <- w875
                          n434 = call "gjson_Parse.vi"("error in"=w891, "JSON String In"=w892, "JSON Cluster"=w889) -> ("error out"=w887:errorcluster, "JSON Cluster Out"=w888:variant)  [unwired: 7 in]
                          n435 = Variant To Data(error in=w887, type=w890, Variant=w888) -> (data=→"data":cluster{"status":string}, error out=w876:errorcluster)
                          "error AURA" <- w876
                          n436 = local read "Report"() -> (w872:string)
                          n437 = call "Reporting_error.vi"("error out 2"=w876, "Concept"="A.U.R.A. Wheel Connection") -> ("Reporting"=w877:string)  [unwired: 1 in]
                          n438 = Concatenate Strings(w877, w874, w874, w875, w874) -> (w873:string)
                          "Report_AURA" <- w873
                          n439 = Concatenate Strings(w873, w872) -> (w871:string)
                          n440 = local write "Report"(w871) -> ()
                        }
                      }
                    }
                  }
                }
              }
              frame #1 {
                n441 = local read "Archivo\nvalido?"() -> (w958:bool)
                n442 = local read "Bytes libre despues de borrar"() -> (w959:u32)
                n443 = local read "Report_AURA"() -> (w955:string)
                n444 = local read "Max archivos"() -> (w956:u32)
                n445 = local read "Path LOG"() -> (w957:path)
                n446 = local read "LOG.txt"() -> (w952:path)
                n447 = local read "Report"() -> (w954:string)
                n448 = local read "Bytes min libre"() -> (w960:u32)
                n449 = local read "TAGS leidos"() -> (w963:path)
                n450 = File/Directory Info(path=w963) -> (size=w966:i64)  [unwired: 1 in, 6 out]
                n451 = case shown="True" w958 {
                  frame False {
                  }
                  frame True {
                    n452 = local read "Nombre de archivo"() -> (w968:path[])
                    n453 = call "Comprimir_a_1_archivo.vi"("Acel_paths"=w968) -> ("path_Pasada"=→"created path":path)
                  }
                }
                n454 = Greater?(x=w966, y=i64 1000000) -> (0:w964:bool)
                n455 = case shown="True" w964 {
                  tunnel: w963 -> [_ w969]
                  frame False {
                  }
                  frame True {
                    n456 = Delete(path (use dialog)=w969) -> ()  [unwired: 4 in, 3 out]
                  }
                }
                n457 = call "BORRADO_MEJORADO_Gonzalo.vi"("Bytes LIBRE OK"=w959, "Bytes Minimo de Memoria libre"=w960) -> ()  [unwired: 10 in]
                n458 = call "Saving_LOG.vi"("Path"=w952, "Report"=w954, "Report AURA"=w955, "Path Carpeta"=w957, "Nº Archivos Max"=w956) -> ("Report"=w953:string)  [unwired: 9 in, 1 out]
                n459 = local write "Report"(w953) -> ()
              }
            }
            n460 = call <vilib>:"Watchdog Clear.vi"("error in (no error)"=w686, "watchdogID in"=w687) -> ("error out"=w680:errorcluster)  [unwired: 5 in]
            n461 = Merge Errors(w682, w680) -> (w698:errorcluster)
            n462 = Unbundle By Name(w698) -> ("status"=w696:bool)
            n463 = Select(t="TEST", s=w696, f="Espera") -> (s? t:f=w695:string)
          }
          frame "TEST" {
            n464 = flat-sequence {
              tunnel: [w985] -> w972
              tunnel: w974 -> [w985]
              frame #0 {
                n465 = local read "Report"() -> (w986:string)
                n466 = call "Reporting_datetime.vi"() -> ("String"=w984:string)  [unwired: 11 in]
                n467 = Concatenate Strings(w984, "\nSTATUS: ERROR TEST\n\n", w986) -> (w988:string)
                n468 = local write "Report"(w988) -> ()
              }
            }
            n469 = local read "Watchdog config"() -> (w979:T1)
            n470 = Merge Errors(w972, w970) -> (w971:errorcluster)
            n471 = call <vilib>:"Watchdog Configure.vi"("error in (no error)"=w970, "expiration actions"=w979, "timeout (1 sec)"=200.0) -> ("error out"=w980:errorcluster, "watchdogID"=w977:u64)  [unwired: 1 in, 2 out]
            n472 = flat-sequence {
              tunnel: [w998] -> w983
              tunnel: w980 -> [w993]
              tunnel: w971 -> [w1011]
              tunnel: [w994] -> w981
              tunnel: w977 -> [w992]
              tunnel: [w991] -> w976
              tunnel: [w990] -> w975
              frame #0 {
                n473 = Get Date/Time In Seconds() -> (seconds since 1Jan1904=w1005:timestamp)
                n474 = local read "Ultimo TEST"() -> (w1006:timestamp)
                n475 = To Double Precision Float(number=w1005) -> (double precision float=w1007:dbl)
                n476 = Subtract(x=w1007, y=3600.0) -> (x-y=w1009:dbl)
                n477 = To Time Stamp(1:w1009) -> (0:w1010:timestamp)
                n478 = call <vilib>:"Watchdog Whack.vi"("error in (no error)"=w993, "reset watchdog after expire? (F)"=TRUE, "watchdogID in"=w992) -> ("error out"=w990:errorcluster, "watchdogID out"=w991:u64)  [unwired: 2 in, 1 out]
                n479 = In Range and Coerce(upper limit=w1005, x=w1006, lower limit=w1010) -> (In Range?=w1004:bool)  [unwired: 1 out]
                n480 = case shown="False" w1004 {
                  tunnel: w1011 -> [w1021 w1045]
                  tunnel: [w1021 w1045] -> w994
                  frame False {
                    n481 = local read "Timeout ruedas"() -> (w1022:bool)
                    n482 = local read "Aviso no detección"() -> (w1025:string)
                    n483 = local read "Aviso temperatura"() -> (w1024:string)
                    n484 = case shown="True" w1022 {
                      selector: w1022 -> [_ w1042]
                      tunnel: ["\r" w1043] -> w1020
                      frame False {
                      }
                      frame True {
                        w1032 = "\n"
                        n485 = local read "Nº Ruedas 1"() -> (w1039:i32)
                        n486 = local read "NºRuedas 2"() -> (w1034:i32)
                        n487 = call "ErrorRuedas.vi"("Buffer Overflow"=w1042) -> ("error out"=w1044:errorcluster)
                        n488 = Number To Decimal String(number=w1039) -> (decimal integer string=w1037:string)  [unwired: 1 in]
                        n489 = Number To Decimal String(number=w1034) -> (decimal integer string=w1033:string)  [unwired: 1 in]
                        n490 = Concatenate Strings("Error Wheel sensors", "\n", "WS1 (wheels):", w1037, w1032, "WS2 (wheels):", w1033, w1032) -> (w1035:string)
                        n491 = call "Error.vi"("Error con..."=w1035, "error comunicacion 2"=w1044) -> ("String"=w1043:string)
                      }
                    }
                    n492 = local read "DC OK"() -> (w1023:string)
                    n493 = call "Cabecera.vi"() -> ("String"=w1030:string)
                    n494 = call "Adquisicion.vi"("Aviso no detección"=w1025) -> ("String"=w1029:string)
                    n495 = call "Temperatura.vi"("Aviso temperatura"=w1024) -> ("String"=w1028:string)
                    n496 = call "Fuente.vi"("DC OK"=w1023) -> ("String"=w1027:string)
                    n497 = call "FPGA.vi"("error out"=w1021) -> ("String"=w1026:string)
                    n498 = Get Date/Time In Seconds() -> (seconds since 1Jan1904=→"Ultimo TEST":timestamp)
                    n499 = Concatenate Strings(w1030, w1029, w1028, w1027, w1026, w1020) -> (w1014:string)
                    n500 = local read "Report"() -> (w1013:string)
                    n501 = Concatenate Strings(w1014, w1013) -> (w1015:string)
                    n502 = local read "Max archivos"() -> (w1016:u32)
                    n503 = local read "Path LOG"() -> (w1019:path)
                    n504 = local read "LOG.txt"() -> (w1017:path)
                    n505 = call "Saving_LOG.vi"("Path"=w1017, "Report"=w1015, "Report AURA"=w1014, "Path Carpeta"=w1019, "Nº Archivos Max"=w1016) -> ("Report"=w1018:string)  [unwired: 9 in, 1 out]
                    n506 = local write "Report"(w1018) -> ()
                  }
                  frame True {
                  }
                }
                n507 = local read "Fallo fotocelula"() -> (w997:bool)
                n508 = local read "T fuera rango"() -> (w1003:bool)
                n509 = Unbundle By Name(w994) -> ("status"=w995:bool)
                n510 = Compound Arithmetic op=OR(w995, w997) -> (w996:bool)
                n511 = local write "Reset del controlador"(w996) -> ()
                n512 = Select(t="UPS", s=w1003, f="Espera") -> (s? t:f=w1000:string)
                n513 = Select(t="Configuracion", s=w996, f=w1000) -> (s? t:f=w998:string)
              }
            }
            n514 = call <vilib>:"Watchdog Clear.vi"("error in (no error)"=w975, "watchdogID in"=w976) -> ("error out"=w973:errorcluster)  [unwired: 5 in]
          }
          frame "Calibracion" {
            n515 = flat-sequence {
              tunnel: w1060 -> [w1836]
              tunnel: w1059 -> [w1835]
              tunnel: [w1836] -> w1058
              tunnel: [w1835] -> w1057
              frame #0 {
                n516 = local read "Report"() -> (w1832:string)
                n517 = call "Reporting_datetime.vi"() -> ("String"=w1831:string)  [unwired: 11 in]
                n518 = Concatenate Strings(w1831, "\nSTATUS: CALIBRATION\n\n\n", w1832) -> (w1834:string)
                n519 = local write "Report"(w1834) -> ()
              }
            }
            n520 = for {
              N: 5 -> [_]
              shift-right: [w1090] -> w1050
              shift-left: w1058 -> [w1092]
              shift-right: [w1089] -> w1046
              shift-left: w1057 -> [w1091]
              shift-right: [w1087] -> _
              shift-left: "Adquisicion" ("element") -> [w1088]
              shift-right: [w1086] -> _
              shift-left: _ -> [w1084]
              shift-right: [w1082] -> w1052
              shift-left: "" -> [w1081]
              i -> [w1080]
              stop <- w1085 stop-if-true
              n521 = case shown="\"Acel_calib\"" w1088 {
                tunnel: w1092 -> [w1100 w1330 w1535 w1697 w1782]
                tunnel: w1091 -> [w1099 w1329 w1534 w1696 w1781]
                tunnel: [w1098 w1330 w1535 w1697 w1782] -> w1090
                tunnel: [w1097 w1329 w1534 w1696 w1781] -> w1089
                tunnel: ["Acel_calib" ("Concept") "Acel_frequency" ("Concept") "Acel_noise" ("Concept") "Acel_result" ("Concept") "Adquisicion" ("Concept")] -> w1087
                tunnel: [sgl[][] [] w1326 w1533 w1695 sgl[][] []] -> w1086
                tunnel: [TRUE w1325 w1532 w1692 FALSE] -> w1079
                tunnel: w1084 -> [_ _ w1523 w1698 w1792]
                tunnel: ["\n" w1323 w1530 w1688 w1780] -> w1083
                frame "Adquisicion", Default {
                  n522 = flat-sequence {
                    tunnel: w1099 -> [w1122]
                    tunnel: w1100 -> [w1123]
                    tunnel: [w1123] -> w1103
                    tunnel: [w1122] -> w1102
                    tunnel: [w1106] -> w1101
                    tunnel: w1103 -> [w1135]
                    tunnel: w1102 -> [w1134]
                    tunnel: w1101 -> [w1131]
                    tunnel: [w1133] -> w1098
                    tunnel: [w1132] -> w1097
                    frame #0 {
                      w1118 = "Calibration" ("element")
                      w1117 = "c"
                      n523 = Format Date/Time String(time format string (%c)="%Y-%m-%d-%H-%M-%S") -> (date/time string=w1109:string)  [unwired: 2 in]
                      n524 = for {
                        N: 1 -> [_]
                        shift-right: [w1124] -> w1104
                        shift-left: _ -> [w1125]
                        n525 = Add(x=w1125, y=0.001) -> (x+y=w1124:dbl)
                      }
                      n526 = Number To Fractional String(number=w1104) -> (F-format string=w1113:string)  [unwired: 3 out]
                      n527 = Search and Replace String(input string=w1113, search string="." ("replace string (\"\")")) -> (result string=w1111:string)  [unwired: 1 in, 8 out]
                      n528 = for {
                        N: 3 -> [_]
                        shift-right: [w1129] -> w1107
                        shift-left: w1111 -> [w1127]
                        n529 = Search and Replace String(input string=w1127, search string="0", offset=4 ("offset (0)")) -> (result string=w1129:string)  [unwired: 1 in, 7 out]
                      }
                      n530 = Concatenate Strings(w1107, "_" ("replace string (\"\")"), w1109) -> (w1106:string)
                      "date/time string 2" <- w1106
                      n531 = Build Array(w1117, w1118, w1106) -> (w1116:string[])
                      n532 = Build Array(w1117, w1118, w1106, "Calibration_LOG.txt" ("element")) -> (w1120:string[])
                      n533 = Array of Strings to Path(0:w1116) -> (2:w1115:path)  [unwired: 1 out]
                      "Folder" <- w1115
                      n534 = Array of Strings to Path(0:w1120) -> (2:→"calibration log":path)  [unwired: 1 out]
                      n535 = Create Folder(path (use dialog)=w1115) -> ()  [unwired: 2 in, 3 out]
                    }
                    frame #1 {
                      n536 = for {
                        N: 11 -> [_]
                        shift-right: [w1154] -> w1133
                        shift-left: w1135 -> [w1164]
                        shift-right: [w1157] -> w1132
                        shift-left: w1134 -> [w1163]
                        tunnel: w1131 -> [w1150]
                        i -> [w1160]
                        n537 = xnode "Invoke Method"("FPGA VI Reference In"=w1164, "error in"=w1163) -> ("FPGA VI Reference Out"=w1162:refnum<k20>, "error out"=w1161:errorcluster)  [unwired: 1 in]
                        n538 = Increment(x=w1160) -> (x+1=w1159:i32)
                        n539 = Number To Decimal String(number=w1159) -> (decimal integer string=w1158:string)  [unwired: 1 in]
                        n540 = flat-sequence {
                          tunnel: w1162 -> [w1175]
                          tunnel: w1161 -> [w1174]
                          tunnel: w1158 -> [w1173]
                          tunnel: [w1175] -> w1156
                          tunnel: [w1174] -> w1155
                          tunnel: [w1168] -> w1151
                          tunnel: w1150 -> [w1168]
                          tunnel: [w1167] -> w1137
                          tunnel: w1156 -> [w1183]
                          tunnel: w1155 -> [w1182]
                          tunnel: [w1183] -> w1153
                          tunnel: [w1182] -> w1152
                          tunnel: w1151 -> [w1180]
                          tunnel: [w1180] -> w1149
                          tunnel: [w1179] -> w1138
                          tunnel: w1137 -> [w1179]
                          tunnel: w1153 -> [w1223]
                          tunnel: w1152 -> [w1222]
                          tunnel: w1149 -> [w1201]
                          tunnel: [w1221] -> w1148
                          tunnel: [w1220] -> w1147
                          tunnel: [w1194] -> w1146
                          tunnel: [w1193] -> w1145
                          tunnel: [w1192] -> w1144
                          tunnel: [w1191] -> w1143
                          tunnel: w1138 -> [w1184]
                          tunnel: w1148 -> [w1250]
                          tunnel: w1147 -> [w1251]
                          tunnel: w1146 -> [w1247]
                          tunnel: w1145 -> [w1246]
                          tunnel: w1144 -> [w1245]
                          tunnel: w1143 -> [w1244]
                          tunnel: [w1249] -> w1142
                          tunnel: [w1241] -> w1141
                          tunnel: [w1238] -> w1140
                          tunnel: [w1237] -> w1139
                          tunnel: [w1313] -> w1157
                          tunnel: [w1314] -> w1154
                          tunnel: w1142 -> [w1319]
                          tunnel: w1141 -> [w1318]
                          tunnel: w1140 -> [w1316]
                          tunnel: w1139 -> [w1315]
                          frame #0 {
                            w1165 = dbl[] [] ("mean")
                            n541 = local read "Report"() -> (w1170:string)
                            n542 = local write "mean"(w1165) -> ()
                            n543 = local write "median"(w1165) -> ()
                            n544 = local write "max"(w1165) -> ()
                            n545 = local write "min"(w1165) -> ()
                            n546 = local write "Value to compare"(w1165) -> ()
                            n547 = Concatenate Strings("\nAcquiring file: ", w1173, "/11\n" ("string"), w1170) -> (w1169:string)
                            n548 = for {
                              N: 1 -> [_]
                              shift-right: [w1176] -> w1167
                              shift-left: _ -> [w1177]
                              n549 = Add(x=w1177, y=0.001) -> (x+y=w1176:dbl)
                            }
                            n550 = local write "Report"(w1169) -> ()
                          }
                          frame #1 {
                            n551 = Wait (ms)(milliseconds to wait=u32 1000) -> ()  [unwired: 1 out]
                          }
                          frame #2 {
                            n552 = local read "Frecuencia de muestreo y módulo CRIO"() -> (w1219:T2)
                            n553 = local read "Frecuencia de muestreo (Hz)"() -> (w1217:dbl)
                            n554 = Number To Fractional String(number=w1184) -> (F-format string=w1198:string)  [unwired: 3 out]
                            n555 = local read "Escaneos de la FIFO por canal"() -> (w1216:u32)
                            n556 = xnode "Read/Write Control"("FPGA VI Reference In"=w1223, "error in"=w1222, "Fotocélula"=TRUE ("Adquirir")) -> ("FPGA VI Reference Out"=w1227:refnum<k20>, "error out"=w1226:errorcluster)
                            n557 = local read "Nº de acelerómetros"() -> (w1214:i32)
                            n558 = local read "Count(mSec)"() -> (w1218:u32)
                            n559 = local read "Nº inductivos"() -> (w1215:i32)
                            n560 = Search and Replace String(input string=w1198, search string="." ("replace string (\"\")")) -> (result string=w1196:string)  [unwired: 1 in, 8 out]
                            n561 = for {
                              N: 3 -> [_]
                              shift-right: [w1235] -> w1199
                              shift-left: w1196 -> [w1233]
                              n562 = Search and Replace String(input string=w1233, search string="0", offset=4 ("offset (0)")) -> (result string=w1235:string)  [unwired: 1 in, 7 out]
                            }
                            n563 = xnode "Read/Write Control"("FPGA VI Reference In"=w1227, "error in"=w1226, "Data Rate"=w1219, "Digital?"=TRUE, "Count(mSec)"=w1218) -> ("FPGA VI Reference Out"=w1229:refnum<k20>, "error out"=w1228:errorcluster)
                            n564 = Format Date/Time String(time format string (%c)="%Y-%m-%d-%H-%M-%S") -> (date/time string=w1200:string)  [unwired: 2 in]
                            n565 = Add(x=w1215, y=w1214) -> (x+y=w1213:i32)
                            n566 = call "DMACalc.vi"("Number of Channels"=w1213, "Number of Samples"=w1216, "Rate (Hz)"=w1217) -> ("Block Size"=w1193:u32, "Time to Acquire Block (ms)"=w1194:i32, "Host Buffer Size"=w1212:u32)  [unwired: 6 in]
                            n567 = xnode "Invoke Method"("FPGA VI Reference In"=w1229, "error in"=w1228, "Requested Depth"=w1212) -> ("FPGA VI Reference Out"=w1231:refnum<k20>, "error out"=w1230:errorcluster)  [unwired: 1 out]
                            n568 = Concatenate Strings(w1199, "_" ("replace string (\"\")"), w1200, ".bin" ("string")) -> (w1207:string)
                            n569 = Build Array("c", "Calibration" ("element"), w1201, w1207) -> (w1206:string[])
                            n570 = xnode "Invoke Method"("FPGA VI Reference In"=w1231, "error in"=w1230) -> ("FPGA VI Reference Out"=w1221:refnum<k20>, "error out"=w1220:errorcluster)
                            n571 = local read "Report"() -> (w1186:string)
                            n572 = Array of Strings to Path(0:w1206) -> (2:w1187:path)  [unwired: 1 out]
                            n573 = Path To String(path=w1187) -> (string=w1190:string)
                            n574 = Get Date/Time In Seconds() -> (seconds since 1Jan1904=→"Inicio pasada 2":timestamp)
                            n575 = Concatenate Strings("\nFile created: ", w1190, "\n", w1186) -> (w1185:string)
                            n576 = Open/Create/Replace File(file path (use dialog)=w1187, operation (0:open)=T4."replace or create", access (0:read/write)=enum16{"read/write", "read-only", "write-only"}."read/write", disable buffering (F)=TRUE) -> (refnum out=w1192:refnum<file>, error out=w1191:errorcluster)  [unwired: 1 in, 2 out]
                            n577 = local write "Report"(w1185) -> ()
                          }
                          frame #3 {
                            n578 = while "Data Acquisition" {
                              tunnel: w1250 -> [w1276]
                              shift-right: [w1283] -> _
                              shift-left: u32 0 ("t") -> [w1279]
                              tunnel: w1247 -> [w1284]
                              tunnel: w1246 -> [w1282]
                              shift-right: [w1285] -> w1241
                              shift-left: w1251 -> [w1275]
                              tunnel: [w1280] -> w1249
                              tunnel: w1245 -> [w1265]
                              tunnel: [w1266] -> w1238
                              shift-right: [w1264] -> w1237
                              shift-left: w1244 -> [w1273]
                              stop <- w1281 stop-if-true
                              # "Detector de presencia"
                              # "Mide el tiempo de paso del tren y con ello se puede calcular\nla velocidad la unidad"
                              n579 = xnode "Invoke Method"("FPGA VI Reference In"=w1276, "error in"=w1275, "Number of Elements"=w1279, "Timeout (ms)"=0) -> ("FPGA VI Reference Out"=w1263:refnum<k20>, "error out"=w1262:errorcluster, "Data"=w1274:fxp<+/-,24,4>[], "Elements Remaining"=w1277:u32)
                              n580 = case "Data Ready" shown="0" w1279 {
                                tunnel: w1284 -> [w1290 _]
                                tunnel: [w1289 u32 0 ("t")] -> w1283
                                tunnel: w1282 -> [w1291 _]
                                tunnel: w1277 -> [w1288 _]
                                tunnel: w1274 -> [_ w1301]
                                tunnel: w1273 -> [w1287 w1303]
                                tunnel: [w1287 w1302] -> w1264
                                tunnel: w1265 -> [w1286 w1300]
                                tunnel: [w1286 w1299] -> w1266
                                frame 0 {
                                n581 = Greater Or Equal?(x=w1288, y=w1291) -> (x >= y?=w1292:bool)
                                n582 = case shown="False" w1292 {
                                tunnel: [u32 0 ("Block Size") w1296] -> w1289
                                tunnel: [w1295 0 ("t")] -> w1293
                                tunnel: w1290 -> [w1295 _]
                                tunnel: w1291 -> [_ w1296]
                                frame False {
                                }
                                frame True {
                                }
                                }
                                n583 = call "WaitMinTimeBetweenCall.vi"("Minimum ms between calls"=w1293) -> ()  [unwired: 2 in]
                                }
                                frame Default {
                                n584 = To Single Precision Float(number=w1301) -> (single precision float=w1298:sgl[])
                                n585 = Write to Binary File(file (use dialog)=w1300, data=w1298, error in=w1303, 5:FALSE ("prepend array or string size? (T)"), 9:T5."little-endian" ("byte order (0:big-endian, network order)")) -> (refnum out=w1299:refnum<file>, error out=w1302:errorcluster)  [unwired: 2 out]
                                }
                              }
                              n586 = local read "Inicio pasada 2"() -> (w1254:timestamp)
                              n587 = Get Date/Time In Seconds() -> (seconds since 1Jan1904=w1255:timestamp)
                              n588 = xnode ("CheckLate")("FPGA VI Reference In"=w1263, "error in"=w1262) -> ("FPGA VI Reference Out"=w1257:refnum<k20>, "error out"=w1271:errorcluster, "Buffer Underflow"=w1252:bool, "Buffer Overflow"=w1253:bool)
                              n589 = To Double Precision Float(number=w1255) -> (double precision float=w1260:dbl)
                              n590 = To Double Precision Float(number=w1254) -> (double precision float=w1261:dbl)
                              n591 = Subtract(x=w1260, y=w1261) -> (x-y=w1268:dbl)
                              "Acquiring time" <- w1268
                              n592 = local write "Buffer Overflow"(w1253) -> ()
                              n593 = local write "Buffer Underflow"(w1252) -> ()
                              n594 = Greater?(x=w1268, y=1.0 ("Tiempo de adquisición")) -> (0:w1259:bool)
                              n595 = call "ErrorOverFlow.vi"("Buffer Overflow"=w1253) -> ("error out"=w1269:errorcluster)
                              n596 = call "ErrorUnderFlow.vi"("Buffer Overflow"=w1252) -> ("error out"=w1270:errorcluster)
                              n597 = Merge Errors(w1271, w1270, w1269) -> (w1258:errorcluster)
                              n598 = Unbundle By Name(w1264) -> ("status"=w1267:bool)
                              n599 = Unbundle By Name(w1258) -> ("status"=w1272:bool)
                              n600 = Compound Arithmetic op=OR(w1272, w1259, w1267) -> (w1281:bool)
                              n601 = case "Flush" shown="True" w1281 {
                                tunnel: w1257 -> [w1307 w1312]
                                tunnel: w1258 -> [w1308 w1311]
                                tunnel: [w1308 w1310] -> w1285
                                tunnel: [w1307 w1309] -> w1280
                                frame False {
                                }
                                frame True {
                                n602 = xnode "Invoke Method"("FPGA VI Reference In"=w1312, "error in"=w1311) -> ("FPGA VI Reference Out"=w1309:refnum<k20>, "error out"=w1310:errorcluster)
                                }
                              }
                            }
                            n603 = call "Reporting_error.vi"("error out 2"=w1241, "Concept"="FPGA ") -> ("Reporting"=w1243:string)  [unwired: 1 in]
                            n604 = local read "Report"() -> (w1240:string)
                            n605 = Concatenate Strings(w1243, w1240) -> (w1242:string)
                            n606 = local write "Report"(w1242) -> ()
                          }
                          frame #4 {
                            n607 = xnode "Read/Write Control"("FPGA VI Reference In"=w1319, "error in"=w1318, "Stop"=TRUE) -> ("FPGA VI Reference Out"=w1320:refnum<k20>, "error out"=w1321:errorcluster)
                            n608 = xnode "Invoke Method"("FPGA VI Reference In"=w1320, "error in"=w1321) -> ("FPGA VI Reference Out"=w1314:refnum<k20>, "error out"=w1313:errorcluster)
                            n609 = Close File(refnum=w1316, error in=w1315) -> ()  [unwired: 2 out]
                          }
                        }
                      }
                    }
                  }
                }
                frame "Acel_calib" {
                  n610 = local read "Folder"() -> (w1332:path)
                  n611 = local read "Frecuencia de muestreo (Hz)"() -> (w1338:dbl)
                  n612 = local read "Nº de acelerómetros"() -> (w1333:i32)
                  n613 = local read "Nº inductivos"() -> (w1334:i32)
                  n614 = local read "Pattern frequency (Hz)"() -> (w1339:dbl)
                  n615 = call <vilib>:"Recursive File List.vi"("Folder Path"=w1332) -> ("All Files in Dir"=w1337:path[])  [unwired: 6 in, 4 out]
                  n616 = Array Size(array=w1337) -> (size(s)=→"Nº meas":i32)
                  n617 = Add(x=w1334, y=w1333) -> (x+y=w1336:i32)
                  n618 = flat-sequence {
                    tunnel: w1337 -> [w1349]
                    tunnel: [w1349] -> w1345
                    tunnel: [w1348] -> w1344
                    tunnel: w1336 -> [w1348]
                    tunnel: [w1347] -> w1343
                    tunnel: w1338 -> [w1347]
                    tunnel: [w1346] -> w1342
                    tunnel: w1339 -> [w1346]
                    tunnel: [w1356] -> w1341
                    tunnel: [w1355] -> w1340
                    tunnel: w1345 -> [w1357]
                    tunnel: w1344 -> [w1354]
                    tunnel: w1343 -> [w1353]
                    tunnel: w1342 -> [w1352]
                    tunnel: [w1351] -> w1322
                    tunnel: w1341 -> [w1469]
                    tunnel: w1340 -> [w1453]
                    tunnel: [w1451] -> w1326
                    tunnel: [TRUE] -> w1325
                    tunnel: [w1484] -> w1323
                    tunnel: [w1459] -> w1324
                    tunnel: w1322 -> [w1454]
                    frame #0 {
                      "Valid\nindex" <- i32[] []
                    }
                    frame #1 {
                      n619 = for {
                        tunnel: w1357 -> [w1379] mode=indexing
                        tunnel: [w1369] -> w1356 mode=indexing
                        tunnel: [w1361] -> w1355 mode=indexing
                        tunnel: w1354 -> [w1367]
                        tunnel: w1353 -> [w1366]
                        tunnel: w1352 -> [w1365]
                        tunnel: [w1359] -> w1351 mode=indexing
                        n620 = Read from Binary File(5:sgl 1.25, 9:T5."little-endian" ("byte order (0:big-endian, network order)"), 10:-1 ("count (1)"), 11:w1379) -> (2:w1380:sgl[])  [unwired: 1 in, 4 out]
                        n621 = case shown="10" w1367 {
                          tunnel: [w1397 w1410 w1420] -> w1361
                          tunnel: w1380 -> [w1398 w1408 w1421]
                          frame 9, Default {
                            n622 = Decimate 1D Array(w1398) -> (w1399:sgl[], w1407:sgl[], w1406:sgl[], w1402:sgl[], w1401:sgl[], w1403:sgl[], w1404:sgl[], w1405:sgl[], w1400:sgl[])
                            n623 = Build Array(w1399, w1407, w1406, w1402, w1401, w1403, w1404, w1405, w1400) -> (w1397:sgl[][])
                          }
                          frame 10 {
                            n624 = Decimate 1D Array(w1408) -> (w1409:sgl[], w1419:sgl[], w1418:sgl[], w1414:sgl[], w1413:sgl[], w1415:sgl[], w1416:sgl[], w1417:sgl[], w1412:sgl[], w1411:sgl[])
                            n625 = Build Array(w1409, w1419, w1418, w1414, w1413, w1415, w1416, w1417, w1412, w1411) -> (w1410:sgl[][])
                          }
                          frame 5 {
                            n626 = Decimate 1D Array(w1421) -> (w1422:sgl[], w1426:sgl[], w1425:sgl[], w1424:sgl[], w1423:sgl[])
                            n627 = Build Array(w1422, w1426, w1425, w1424, w1423) -> (w1420:sgl[][])
                          }
                        }
                        n628 = Array Size(array=w1361) -> (size(s)=w1360:i32[])
                        n629 = Index Array(array=w1360, index=1) -> (element=w1359:i32)
                        n630 = for {
                          tunnel: w1361 -> [w1429] mode=indexing
                          tunnel: [w1432] -> w1376 mode=indexing
                          tunnel: w1366 -> [w1431]
                          tunnel: w1365 -> [w1430]
                          n631 = call-poly <vilib>:"Basic Averaged DC-RMS.vi"("signal in"=w1429) -> ("DC value"=w1442:dbl)  [unwired: 7 in, 3 out]
                          n632 = Array Size(array=w1429) -> (size(s)=→"size(s) 3":i32)
                          n633 = Subtract(x=w1429, y=w1442) -> (x-y=w1438:dbl[])
                          n634 = Divide(x=w1431, y=w1430) -> (x/y=w1439:dbl)
                          n635 = Array Size(array=w1438) -> (size(s)=w1440:i32)
                          n636 = Subtract(x=w1440, y=w1439) -> (x-y=w1441:dbl)
                          n637 = for {
                            N: w1441 -> [_]
                            tunnel: w1439 -> [w1444]
                            tunnel: [w1447] -> w1427 mode=indexing
                            tunnel: w1438 -> [w1446]
                            i -> [w1445]
                            n638 = Array Subset(array=w1446, index=w1445, length=w1444) -> (w1443:dbl[])
                            n639 = call-poly <vilib>:"RMS.vi"("X"=w1443) -> ("rms value"=w1447:dbl)  [unwired: 1 out]
                          }
                          n640 = Greater?(x=w1427, y=0.004 ("threshold y")) -> (0:w1436:bool[])
                          n641 = Search 1D Array(1D array=w1436, element=TRUE) -> (index of element=w1434:i32)  [unwired: 1 in]
                          n642 = Not Equal?(x=w1434, y=-1) -> (x != y?=w1432:bool)
                        }
                        n643 = Array Size(array=w1361) -> (size(s)=→"size(s)":i32[])
                        n644 = while {
                          tunnel: w1376 -> [w1396]
                          shift-right: [w1388] -> _
                          shift-left: 0 ("index of element") -> [w1393]
                          shift-right: [w1389] -> w1368
                          shift-left: 0 ("index of element") -> [w1390]
                          tunnel: [w1387] -> w1364 mode=indexing
                          i -> [w1391]
                          stop <- w1394 stop-if-true
                          n645 = Add(x=w1390, y=w1391) -> (x+y=w1389:i32)
                          n646 = Search 1D Array(1D array=w1396, element=TRUE, start index (0)=w1393) -> (index of element=w1387:i32)
                          n647 = Equal?(x=w1387, y=-1) -> (x = y?=w1394:bool)
                          n648 = Increment(x=w1387) -> (x+1=w1388:i32)
                        }
                        n649 = Delete From Array(array=w1364, length=1) -> (array with subset deleted=w1363:i32[])  [unwired: 1 in, 1 out]
                        n650 = Array Size(array=w1363) -> (size(s)=w1372:i32)
                        n651 = Equal?(x=w1368, y=1) -> (x = y?=w1371:bool)
                        n652 = Equal?(x=w1372, y=1) -> (x = y?=w1370:bool)
                        n653 = And(x=w1370, y=w1371) -> (x .and. y?=w1369:bool)
                        n654 = case shown="False" w1369 {
                          tunnel: w1363 -> [_ w1386]
                          frame False {
                          }
                          frame True {
                            n655 = local read "Valid\nindex"() -> (w1384:i32[])
                            n656 = Insert Into Array(array=w1384, new element=w1386) -> (w1385:i32[])  [unwired: 1 in]
                            n657 = local write "Valid\nindex"(w1385) -> ()
                          }
                        }
                      }
                    }
                    frame #2 {
                      w1468 = 0 ("index of element")
                      (unwired) 0 ("index of element")
                      n658 = local read "Valid\nindex"() -> (w1474:i32[])
                      n659 = Array Max & Min(array=w1454) -> (min value=w1450:i32)  [unwired: 3 out]
                      n660 = Delete From Array(array=w1453, index (dim 1)="Accelerometer") -> (deleted portion=w1452:sgl[][])  [unwired: 3 in, 1 out]
                      n661 = Sort 1D Array(array=w1474) -> (sorted array=w1470:i32[])
                      "sorted array" <- w1470
                      n662 = Array Subset(array=w1452, index (col)=0 ("index"), length (col)=w1450) -> (w1451:sgl[][])  [unwired: 2 in]
                      n663 = for {
                        tunnel: w1470 -> [w1505] mode=indexing
                        shift-right: [w1505] -> _
                        shift-left: -1 ("y") -> [w1506]
                        tunnel: [w1505] -> w1479 mode=indexing if=w1504
                        shift-right: [w1501] -> _
                        shift-left: 0 ("y") -> [w1502]
                        tunnel: [w1501] -> w1477 mode=indexing
                        n664 = Not Equal?(x=w1505, y=w1506) -> (x != y?=w1504:bool)
                        n665 = Increment(x=w1502) -> (x+1=w1503:i32)
                        n666 = Select(t=1 ("y"), s=w1504, f=w1503) -> (s? t:f=w1501:i32)
                      }
                      "Array" <- w1479
                      "Array 3" <- w1477
                      n667 = for {
                        tunnel: w1469 -> [w1511] mode=indexing
                        shift-right: [w1510] -> _
                        shift-left: w1453 -> [w1512]
                        shift-right: [w1507] -> _
                        shift-left: 0 ("index of element") -> [w1508]
                        i -> [w1509]
                        n668 = case shown="False" w1511 {
                          tunnel: w1512 -> [w1518 w1520]
                          tunnel: [w1517 w1520] -> w1510
                          tunnel: w1509 -> [w1516 _]
                          tunnel: w1508 -> [w1513 w1519]
                          tunnel: [w1514 w1519] -> w1507
                          frame False {
                            n669 = Subtract(x=w1516, y=w1513) -> (x-y=w1515:i32)
                            n670 = Delete From Array(array=w1518, index (dim 0)=w1515) -> (array with subset deleted=w1517:sgl[][][])  [unwired: 3 in, 1 out]
                            n671 = Increment(x=w1513) -> (x+1=w1514:i32)
                          }
                          frame True {
                          }
                        }
                      }
                      n672 = Array Max & Min(array=w1477) -> (max value=→"max value":i32, max index (indices)=w1475:i32)  [unwired: 2 out]
                      "max index(es)" <- w1475
                      n673 = Array Size(array=w1451) -> (size(s)=→"size(s) 2":i32[])
                      n674 = Index Array(array=w1470, index=w1475) -> (element=w1459:i32)
                      "element" <- w1459
                      n675 = local read "Frecuencia de muestreo (Hz)"() -> (w1457:dbl)
                      n676 = Equal?(x=w1474, y=w1459) -> (x = y?=w1472:bool[])
                      n677 = Boolean To (0,1)(Boolean=w1472) -> (0, 1=w1471:i16[])
                      n678 = Add Array Elements(numeric array=w1471) -> (sum=w1463:i16)
                      n679 = Equal?(x=w1459, y=w1468) -> (x = y?=w1466:bool)
                      n680 = Equal?(x=w1468, y=w1463) -> (x = y?=w1465:bool)
                      n681 = Increment(x=w1459) -> (x+1=w1473:i32)
                      n682 = local read "Nº meas"() -> (w1485:i32)
                      n683 = Not And(1:w1465, 2:w1466) -> (0:w1464:bool)
                      n684 = for {
                        tunnel: w1451 -> [w1499] mode=indexing
                        tunnel: w1457 -> [w1497]
                        tunnel: [w1496] -> w1456 mode=indexing
                        n685 = Reciprocal(x=w1497) -> (1/x=w1498:dbl)
                        n686 = Bundle By Name("Y"=w1499, "dt"=w1498) -> (w1496:waveform(sgl))  [unwired: 1 in]
                      }
                      n687 = Number To Decimal String(number=w1473) -> (decimal integer string=w1461:string)  [unwired: 1 in]
                      n688 = Select(t=w1461, s=w1464, f=" NONE ") -> (s? t:f=w1462:string)
                      n689 = Number To Decimal String(number=w1463) -> (decimal integer string=w1491:string)  [unwired: 1 in]
                      n690 = Number To Decimal String(number=w1485) -> (decimal integer string=w1489:string)  [unwired: 1 in]
                      n691 = Divide(x=w1463, y=w1485) -> (x/y=w1487:dbl)
                      n692 = for {
                        tunnel: w1456 -> [w1495] mode=indexing
                        tunnel: [w1492] -> w1455 mode=concatenating
                        n693 = call "Convert to Dynamic Data"("Waveform"=w1495) -> ("Dynamic Data Type"=w1494:dynamicdata)  [unwired: 3 in]
                        n694 = call "Tone Measurements"("Signals"=w1494) -> ("Frequency"=w1493:dynamicdata)  [unwired: 9 in, 1 out]
                        n695 = call "Convert from Dynamic Data"("Dynamic Data Type"=w1493) -> ("Array"=w1492:dbl[])  [unwired: 3 in]
                      }
                      "Frequency" <- w1455
                      n696 = Greater?(x=w1487, y=0.6) -> ()  [unwired: 1 out]
                      n697 = Concatenate Strings("\nACCELEROMETER DETECTOR:\n\nAccelerometer detected: ", w1462, " \nAccelerometer detected in  ", w1491, " of ", w1489, " measurements\n------------------------------------------------------------------------------------------------------------------------------------------------") -> (w1484:string)
                    }
                  }
                  n698 = local read "Report"() -> (w1327:string)
                  n699 = Concatenate Strings(w1323, w1327) -> (w1328:string)
                  n700 = local write "Report"(w1328) -> ()
                  "Accel.detected" <- w1324
                }
                frame "Acel_frequency" {
                  n701 = local read "Low cutoff freq"() -> (w1525:dbl)
                  n702 = local read "Frequency"() -> (w1526:dbl[])
                  n703 = local read "Frecuencia de muestreo (Hz)"() -> (w1528:dbl)
                  n704 = for {
                    tunnel: w1523 -> [w1559] mode=indexing
                    tunnel: w1528 -> [w1557]
                    tunnel: [w1556] -> w1527 mode=indexing
                    n705 = Reciprocal(x=w1557) -> (1/x=w1558:dbl)
                    n706 = Bundle By Name("Y"=w1559, "dt"=w1558) -> (w1556:waveform(sgl))  [unwired: 1 in]
                  }
                  "Waveform Graph" <- w1527
                  n707 = local read "Pattern frequency (Hz)"() -> (w1529:dbl)
                  n708 = Less?(x=w1526, y=w1525) -> (x < y?=w1521:bool[])
                  n709 = for {
                    tunnel: w1521 -> [w1546] mode=indexing
                    shift-right: [w1545] -> w1522
                    shift-left: w1523 -> [w1547]
                    shift-right: [w1542] -> _
                    shift-left: 0 ("index of element") -> [w1543]
                    i -> [w1544]
                    n710 = case shown="False" w1546 {
                      tunnel: w1547 -> [w1553 w1555]
                      tunnel: [w1552 w1555] -> w1545
                      tunnel: w1544 -> [w1551 _]
                      tunnel: w1543 -> [w1548 w1554]
                      tunnel: [w1549 w1554] -> w1542
                      frame False {
                        n711 = Subtract(x=w1551, y=w1548) -> (x-y=w1550:i32)
                        n712 = Delete From Array(array=w1553, index (row)=w1550) -> (array with subset deleted=w1552:sgl[][])  [unwired: 2 in, 1 out]
                        n713 = Increment(x=w1548) -> (x+1=w1549:i32)
                      }
                      frame True {
                      }
                    }
                  }
                  n714 = flat-sequence {
                    tunnel: w1522 -> [w1566]
                    tunnel: w1528 -> [w1563]
                    tunnel: w1529 -> [w1560]
                    tunnel: [w1568] -> w1541
                    tunnel: [w1562] -> w1540
                    tunnel: [w1561] -> w1539
                    tunnel: [w1560] -> w1538
                    tunnel: w1541 -> [w1645]
                    tunnel: w1540 -> [w1627]
                    tunnel: w1539 -> [w1644]
                    tunnel: w1538 -> [w1643]
                    tunnel: [w1645] -> w1533
                    tunnel: [w1629] -> w1530
                    tunnel: [w1628] -> w1532
                    tunnel: [w1627] -> _
                    frame #0 {
                      n715 = for {
                        tunnel: w1566 -> [w1618] mode=indexing
                        tunnel: w1563 -> [w1617]
                        tunnel: w1560 -> [w1613]
                        tunnel: [w1594] -> w1562 mode=indexing
                        tunnel: [w1588] -> w1561 mode=indexing
                        n716 = Reciprocal(x=w1617) -> (1/x=w1619:dbl)
                        n717 = Bundle By Name("Y"=w1618, "dt"=w1619) -> (w1616:waveform(sgl))  [unwired: 1 in]
                        n718 = call-poly <vilib>:"FFT Spectrum (Mag-Phase).vi"("time signal"=w1616) -> ("magnitude"=w1615:cluster{"f0":dbl, "df":dbl, "magnitude":dbl[]})  [unwired: 6 in, 4 out]
                        n719 = Unbundle By Name(w1615) -> ("magnitude"=w1607:dbl[], "df"=w1589:dbl)
                        n720 = Multiply(x=1.03, y=w1613) -> (x*y=w1610:dbl)
                        n721 = Multiply(x=w1613, y=0.97 ("x")) -> (x*y=w1611:dbl)
                        n722 = Divide(x=w1611, y=w1589) -> (x/y=w1608:dbl)
                        n723 = Divide(x=w1610, y=w1589) -> (x/y=w1605:dbl)
                        n724 = Array Max & Min(array=w1607) -> (max value=w1600:dbl, max index (indices)=w1590:i32)  [unwired: 2 out]
                        n725 = Array Size(array=w1607) -> (size(s)=w1606:i32)
                        n726 = Multiply(x=w1590, y=w1589) -> (x*y=w1588:dbl)
                        n727 = Subtract(x=w1606, y=w1605) -> (x-y=w1604:dbl)
                        n728 = In Range and Coerce(upper limit=w1610, x=w1588, lower limit=w1611) -> (In Range?=w1593:bool)  [unwired: 1 out]
                        n729 = Array Subset(array=w1607, index=w1605, length=w1604) -> (w1603:dbl[])
                        n730 = Array Subset(array=w1607, index=0, length=w1608) -> (w1602:dbl[])
                        n731 = Array Max & Min(array=w1603) -> (max value=w1601:dbl)  [unwired: 3 out]
                        n732 = Array Max & Min(array=w1602) -> (max value=w1599:dbl)  [unwired: 3 out]
                        n733 = Divide(x=w1600, y=w1599) -> (x/y=w1597:dbl)
                        n734 = Divide(x=w1600, y=w1601) -> (x/y=w1598:dbl)
                        n735 = Greater?(x=w1598, y=3.0) -> (0:w1592:bool)
                        n736 = Greater?(x=w1597, y=3.0) -> (0:w1591:bool)
                        n737 = Compound Arithmetic op=AND(w1593, w1592, w1591) -> (w1594:bool)
                      }
                      n738 = for {
                        shift-right: [w1575] -> w1568
                        shift-left: w1566 -> [w1576]
                        tunnel: w1562 -> [w1574] mode=indexing
                        shift-right: [w1571] -> _
                        shift-left: 0 ("index of element") -> [w1572]
                        shift-right: [w1569] -> w1565
                        shift-left: w1561 -> [w1570]
                        i -> [w1573]
                        n739 = case shown="False" w1574 {
                          tunnel: w1576 -> [w1584 w1587]
                          tunnel: [w1583 w1587] -> w1575
                          tunnel: w1573 -> [w1582 _]
                          tunnel: w1572 -> [w1581 w1586]
                          tunnel: [w1580 w1586] -> w1571
                          tunnel: w1570 -> [w1579 w1585]
                          tunnel: [w1577 w1585] -> w1569
                          frame False {
                            n740 = Subtract(x=w1582, y=w1581) -> (x-y=w1578:i32)
                            n741 = Delete From Array(array=w1584, index (row)=w1578) -> (array with subset deleted=w1583:sgl[][])  [unwired: 2 in, 1 out]
                            n742 = Increment(x=w1581) -> (x+1=w1580:i32)
                            n743 = Delete From Array(array=w1579, index=w1578) -> (array with subset deleted=w1577:dbl[])  [unwired: 1 in, 1 out]
                          }
                          frame True {
                          }
                        }
                      }
                      n744 = call <vilib>:"Std Deviation and Variance.vi"("X"=w1565) -> ("mean"=→"Mean\nfrequency":dbl)  [unwired: 1 in, 2 out]
                    }
                    frame #1 {
                      w1624 = "\r"
                      n745 = for {
                        tunnel: w1627 -> [w1653] mode=indexing
                        tunnel: w1644 -> [w1672] mode=indexing
                        tunnel: w1643 -> [w1671]
                        tunnel: [w1654] -> w1641 mode=indexing
                        shift-right: [w1648] -> w1639
                        shift-left: 0 -> [w1649]
                        i -> [w1674]
                        n746 = Increment(x=w1674) -> (x+1=w1673:i32)
                        n747 = Select(t=1, s=w1653, f=0) -> (s? t:f=w1650:i32)
                        n748 = Divide(x=w1672, y=w1671) -> (x/y=w1669:dbl)
                        n749 = Select(t="TRUE", s=w1653, f="FALSE") -> (s? t:f=w1663:string)
                        n750 = Number To Decimal String(number=w1673) -> (decimal integer string=w1666:string)  [unwired: 1 in]
                        n751 = Number To Fractional String(number=w1672, precision (6)=i16 2) -> (F-format string=w1660:string)  [unwired: 2 in]
                        n752 = Add(x=w1650, y=w1649) -> (x+y=w1648:i32)
                        n753 = Greater Than 0?(x=w1669) -> (x > 0?=w1670:bool)
                        n754 = case shown="True" w1670 {
                          tunnel: w1669 -> [w1682 w1684]
                          tunnel: [w1678 w1686] -> w1668
                          tunnel: ["-" " "] -> w1658
                          frame False {
                            n755 = Subtract(x=1.0, y=w1682) -> (x-y=w1680:dbl)
                            n756 = Multiply(x=100.0, y=w1680) -> (x*y=w1678:dbl)
                          }
                          frame True {
                            n757 = Decrement(x=w1684) -> (x-1=w1685:dbl)
                            n758 = Multiply(x=100.0, y=w1685) -> (x*y=w1686:dbl)
                          }
                        }
                        n759 = Number To Fractional String(number=w1668, precision (6)=i16 2) -> (F-format string=w1657:string)  [unwired: 2 in]
                        n760 = Concatenate Strings("\n\nMeasurement: ", w1666, "\r", "Frequency valid: ", w1663, "\r", "Frequency: ", w1660, ", ", w1658, w1657, " % of error in frequency", "\r") -> (w1654:string)
                      }
                      n761 = Array Size(array=w1627) -> (size(s)=w1638:i32)
                      n762 = Number To Decimal String(number=w1638) -> (decimal integer string=w1633:string)  [unwired: 1 in]
                      n763 = Number To Decimal String(number=w1639) -> (decimal integer string=w1625:string)  [unwired: 1 in]
                      n764 = Divide(x=w1639, y=w1638) -> (x/y=w1622:dbl)
                      n765 = Greater?(x=w1622, y=0.8) -> (0:w1628:bool)
                      n766 = Multiply(x=100.0, y=w1622) -> (x*y=w1621:dbl)
                      n767 = Number To Fractional String(number=w1621, precision (6)=i16 2) -> (F-format string=w1632:string)  [unwired: 2 in]
                      n768 = Select(t="OK\n------------------------------------------------------------------------", s=w1628, f="FAIL (REPEAT ACEL CALIBRATION)\n------------------------------------------------------------------------") -> (s? t:f=w1630:string)
                      n769 = Concatenate Strings("FREQUENCY TEST:\n \n- MEASUREMENT OK IF +/- 5% FREQ PATTERN\n\n- FREQUENCY ANALYSYS MORE THAN 80% OF THE MEASUREMENTS INSIDE OF THE RANGE\n", w1641, w1624, w1624, w1625, " measurements OK of ", w1633, " , ", w1632, " %\n\nFREQUENCY ANALYSIS: ", w1630) -> (w1629:string)
                    }
                  }
                  n770 = local read "Report"() -> (w1537:string)
                  n771 = Concatenate Strings(w1530, w1537) -> (w1536:string)
                  n772 = local write "Report"(w1536) -> ()
                }
                frame "Acel_noise" {
                  n773 = local read "Frecuencia de muestreo (Hz)"() -> (w1691:dbl)
                  n774 = local read "Pattern frequency (Hz)"() -> (w1690:dbl)
                  n775 = flat-sequence {
                    tunnel: w1698 -> [w1709]
                    tunnel: [w1725] -> w1695
                    tunnel: w1691 -> [w1724]
                    tunnel: w1690 -> [w1723]
                    tunnel: [w1712] -> w1688
                    tunnel: [w1711] -> w1692
                    frame #0 {
                      n776 = for {
                        tunnel: w1709 -> [w1773] mode=indexing
                        tunnel: [w1766] -> w1729 mode=indexing
                        tunnel: w1724 -> [w1761]
                        tunnel: w1723 -> [w1762]
                        n777 = call-poly <vilib>:"Basic Averaged DC-RMS.vi"("signal in"=w1773) -> ("DC value"=w1774:dbl)  [unwired: 7 in, 3 out]
                        n778 = Subtract(x=w1773, y=w1774) -> (x-y=w1763:dbl[])
                        n779 = Divide(x=w1761, y=w1762) -> (x/y=w1770:dbl)
                        n780 = Array Size(array=w1763) -> (size(s)=w1771:i32)
                        n781 = Subtract(x=w1771, y=w1770) -> (x-y=w1772:dbl)
                        n782 = for {
                          N: w1772 -> [_]
                          tunnel: w1770 -> [w1776]
                          tunnel: [w1779] -> w1764 mode=indexing
                          tunnel: w1763 -> [w1778]
                          i -> [w1777]
                          n783 = Array Subset(array=w1778, index=w1777, length=w1776) -> (w1775:dbl[])
                          n784 = call-poly <vilib>:"RMS.vi"("X"=w1775) -> ("rms value"=w1779:dbl)  [unwired: 1 out]
                        }
                        n785 = Array Max & Min(array=w1764) -> (max value=w1768:dbl, min value=w1767:dbl)  [unwired: 2 out]
                        n786 = call <vilib>:"Std Deviation and Variance.vi"("X"=w1764) -> ("mean"=w1765:dbl)  [unwired: 1 in, 2 out]
                        n787 = call <vilib>:"Median.vi"("X"=w1764) -> ("median"=w1769:dbl)  [unwired: 1 out]
                        n788 = Build Array(w1765, w1769, w1768, w1767) -> (w1766:dbl[])
                      }
                      n789 = Multiply(x=w1729, y=1000 ("median")) -> (x*y=w1708:dbl[][])
                      n790 = Index Array(array=w1708, index (col) #1=0 ("disabled index (col)"), index (col) #2=1 ("index (col)"), index (col) #3=2 ("index (col)"), index (col) #4=3 ("index (col)")) -> (element #1=→"mean":dbl[], element #2=→"median":dbl[], element #3=→"max":dbl[], element #4=→"min":dbl[])  [unwired: 4 in]
                      n791 = for {
                        tunnel: w1708 -> [w1756] mode=indexing
                        tunnel: [w1753] -> w1710 mode=indexing
                        tunnel: [w1751] -> w1699 mode=indexing
                        (unwired) 0.2 ("x")
                        n792 = local read "noise_range"() -> (w1752:dbl)
                        n793 = call <vilib>:"Median.vi"("X"=w1756) -> ("median"=w1751:dbl)  [unwired: 1 out]
                        n794 = Subtract(x=w1751, y=w1752) -> (x-y=w1754:dbl)
                        n795 = Add(x=w1752, y=w1751) -> (x+y=w1755:dbl)
                        n796 = for {
                          tunnel: w1756 -> [w1760] mode=indexing
                          tunnel: w1755 -> [w1759]
                          tunnel: w1754 -> [w1758]
                          tunnel: [w1757] -> w1753 mode=indexing
                          n797 = In Range and Coerce(upper limit=w1759, x=w1760, lower limit=w1758) -> (In Range?=w1757:bool)  [unwired: 1 out]
                        }
                      }
                      "Value to compare" <- w1699
                      n798 = for {
                        tunnel: w1710 -> [w1750] mode=indexing
                        tunnel: [w1749] -> w1726 mode=indexing
                        n799 = And Array Elements(Boolean array=w1750) -> (logical AND=w1749:bool)
                      }
                      n800 = for {
                        shift-right: [w1736] -> w1725
                        shift-left: w1709 -> [w1737]
                        tunnel: w1726 -> [w1735] mode=indexing
                        shift-right: [w1732] -> w1722
                        shift-left: 0 ("index of element") -> [w1733]
                        shift-right: [w1730] -> w1717
                        shift-left: 0 ("index of element") -> [w1731]
                        i -> [w1734]
                        n801 = case shown="False" w1735 {
                          tunnel: w1737 -> [w1744 w1748]
                          tunnel: [w1743 w1748] -> w1736
                          tunnel: w1734 -> [w1742 _]
                          tunnel: w1733 -> [w1741 w1747]
                          tunnel: [w1740 w1747] -> w1732
                          tunnel: w1731 -> [w1738 w1746]
                          tunnel: [w1738 w1745] -> w1730
                          frame False {
                            n802 = Subtract(x=w1742, y=w1741) -> (x-y=w1739:i32)
                            n803 = Delete From Array(array=w1744, index (row)=w1739) -> (array with subset deleted=w1743:sgl[][])  [unwired: 2 in, 1 out]
                            n804 = Increment(x=w1741) -> (x+1=w1740:i32)
                          }
                          frame True {
                            n805 = Increment(x=w1746) -> (x+1=w1745:i32)
                          }
                        }
                      }
                      n806 = Number To Decimal String(number=w1722) -> (decimal integer string=w1720:string)  [unwired: 1 in]
                      n807 = Greater?(x=w1717, y=3) -> (0:w1711:bool)
                      n808 = Select(t="------------------------------------------------------------------------", s=w1711, f="There are not enough correct measurements to calibrate\n\nREPEAT THE ACCELEROMETER CALIBRATION\n------------------------------------------------------------------------") -> (s? t:f=w1713:string)
                      n809 = Concatenate Strings("SIGNAL NOISE ANALYSIS:\n\nFiles erasing by  noise: ", w1720, "\r", w1713) -> (w1712:string)
                    }
                  }
                  n810 = local read "Report"() -> (w1693:string)
                  n811 = Concatenate Strings(w1688, w1693) -> (w1694:string)
                  n812 = local write "Report"(w1694) -> ()
                }
                frame "Acel_result" {
                  n813 = local read "Frecuencia de muestreo (Hz)"() -> (w1791:dbl)
                  n814 = local read "Pattern frequency (Hz)"() -> (w1790:dbl)
                  n815 = local read "Pattern amplitude (g)"() -> (w1789:dbl)
                  n816 = flat-sequence {
                    tunnel: w1792 -> [w1810]
                    tunnel: w1791 -> [w1808]
                    tunnel: w1790 -> [w1807]
                    tunnel: w1789 -> [w1806]
                    tunnel: [w1805] -> w1785
                    tunnel: [w1796] -> _
                    tunnel: [w1795] -> w1780
                    frame #0 {
                      n817 = for {
                        tunnel: w1810 -> [w1824] mode=indexing
                        tunnel: w1808 -> [w1820]
                        tunnel: w1807 -> [w1817]
                        tunnel: [w1818] -> w1815 mode=indexing
                        n818 = call-poly <vilib>:"Basic Averaged DC-RMS.vi"("signal in"=w1824) -> ("DC value"=w1825:dbl)  [unwired: 7 in, 3 out]
                        n819 = Subtract(x=w1824, y=w1825) -> (x-y=w1816:dbl[])
                        n820 = Divide(x=w1820, y=w1817) -> (x/y=w1821:dbl)
                        n821 = Array Size(array=w1816) -> (size(s)=w1822:i32)
                        n822 = Subtract(x=w1822, y=w1821) -> (x-y=w1823:dbl)
                        n823 = for {
                          N: w1823 -> [_]
                          tunnel: w1821 -> [w1827]
                          tunnel: [w1830] -> w1819 mode=indexing
                          tunnel: w1816 -> [w1829]
                          i -> [w1828]
                          n824 = Array Subset(array=w1829, index=w1828, length=w1827) -> (w1826:dbl[])
                          n825 = call-poly <vilib>:"RMS.vi"("X"=w1826) -> ("rms value"=w1830:dbl)  [unwired: 1 out]
                        }
                        n826 = call <vilib>:"Std Deviation and Variance.vi"("X"=w1819) -> ("mean"=w1818:dbl)  [unwired: 1 in, 2 out]
                      }
                      n827 = call <vilib>:"Std Deviation and Variance.vi"("X"=w1815) -> ("mean"=w1814:dbl)  [unwired: 1 in, 2 out]
                      n828 = Divide(x=w1806, y=w1814) -> (x/y=w1812:dbl)
                      n829 = Reciprocal(x=w1812) -> (1/x=w1809:dbl)
                      n830 = Multiply(x=w1809, y=1000.0) -> (x*y=w1802:dbl)
                      n831 = Number To Fractional String(number=w1802, precision (6)=i16 2) -> (F-format string=w1798:string)  [unwired: 2 in]
                      n832 = Divide(x=w1809, y=9.81) -> (x/y=w1805:dbl)
                      n833 = In Range and Coerce(upper limit=11.5, x=w1802, lower limit=8.5) -> (In Range?=w1796:bool)  [unwired: 1 out]
                      n834 = Select(t="\n\nACCELEROMETER CALIBRATED CORRECTLY\n------------------------------------------------------------------------ \n", s=w1796, f="\n\nCALIBRATION FAILED\nSENSITIVITY OUT OF RANGE (8,5-11,5)\n------------------------------------------------------------------------ \n") -> (s? t:f=w1797:string)
                      n835 = Concatenate Strings("\nAMPLITUDE CALIBRATION:\n\nSENSIVITY: ", w1798, w1797, "\r") -> (w1795:string)
                    }
                  }
                  n836 = local read "Report"() -> (w1788:string)
                  n837 = Concatenate Strings(w1780, w1788) -> (w1787:string)
                  n838 = local write "Report"(w1787) -> ()
                  "Calibration parameter" <- w1785
                }
              }
              n839 = Not(x=w1079) -> (.not. x?=w1085:bool)
              n840 = Concatenate Strings(w1081, w1083) -> (w1082:string)
              "Numeric" <- w1080
            }
            n841 = local read "calibration log"() -> (w1051:path)
            n842 = Write to Text File(file (use dialog)=w1051, text=w1052) -> ()  [unwired: 2 in, 3 out]
            n843 = flat-sequence {
              tunnel: w1050 -> [w1066]
              tunnel: w1046 -> [w1065]
              tunnel: [w1066] -> w1049
              tunnel: [w1065] -> w1047
              frame #0 {
                # "Antes Accel. detected"
                n844 = local read "Accelerometer"() -> (w1061:i32)
                n845 = local read "Save calibration"() -> (w1064:bool)
                n846 = Add(x=w1061, y=8) -> (x+y=w1063:i32)
                n847 = case shown="True" w1064 {
                  tunnel: w1063 -> [_ w1067]
                  frame False {
                  }
                  frame True {
                    w1077 = "Parametros"  # Key 1
                    n848 = local read "configuration file path"() -> (w1069:path)
                    n849 = local read "Calibration parameter"() -> (w1068:dbl)
                    n850 = Number To Decimal String(number=w1067) -> (decimal integer string=w1078:string)  [unwired: 1 in]
                    n851 = Concatenate Strings(w1077, w1078) -> (w1071:string)
                    n852 = call <vilib>:"Open Config Data.vi"("create file if necessary (T)"=TRUE, "configuration file path"=w1069) -> ("error out"=w1072:errorcluster, "refnum"=w1073:T12)  [unwired: 1 in, 7 out]
                    n853 = call-poly <vilib>:"Write Key.vi"("section"="Adquisicion", "error in (no error)"=w1072, "value"=w1068, "key"=w1071, "refnum"=w1073) -> ("error out"=w1076:errorcluster, "refnum out"=w1075:T12)  [unwired: 3 in, 2 out]
                    n854 = call <vilib>:"Close Config Data.vi"("error in (no error)"=w1076, "refnum"=w1075) -> ()  [unwired: 8 in, 2 out]
                  }
                }
              }
            }
          }
          frame "UPS" {
            n855 = flat-sequence {
              tunnel: w1839 -> [w1850]
              tunnel: [w1850] -> w1838
              frame #0 {
                n856 = local read "Report"() -> (w1849:string)
                n857 = call "Reporting_datetime.vi"() -> ("String"=w1847:string)  [unwired: 11 in]
                n858 = Concatenate Strings(w1847, "\nSTATUS: UPS\n\n", w1849) -> (w1848:string)
                n859 = local write "Report"(w1848) -> ()
              }
            }
            n860 = node-c288() -> (w1845:T6)  [unwired: 4 in]
            n861 = timed-loop {
              timing: w1845 -> [_]
              timing-out: [_] -> w1844
              tunnel: w1837 -> [w1859]
              tunnel: w1838 -> [w1858]
              tunnel: [w1857] -> w1843
              tunnel: [w1856] -> w1842
              stop <- w1851 stop-if-true
              n862 = node-c288() -> ()  [unwired: 1 in, 1 out]
              n863 = xnode "Read/Write Control"("FPGA VI Reference In"=w1859, "error in"=w1858) -> ("FPGA VI Reference Out"=w1857:refnum<k20>, "error out"=w1856:errorcluster, "DC OK"=w1854:bool, "Chassis Temperature"=w1855:i16)
              n864 = call "ControlTemperatura.vi"("Chassis Temperature"=w1855) -> ("T fuera rango"=w1853:bool)  [unwired: 2 out]
              n865 = Not(x=w1853) -> (.not. x?=w1852:bool)
              n866 = And(x=w1854, y=w1852) -> (x .and. y?=w1851:bool)
              n867 = node-c288() -> ()  [unwired: 1 in, 1 out]
            }
            n868 = node-c288(w1844) -> ()  [unwired: 1 out]
          }
        }
        "error manipulacion archivos" <- w112
        n869 = local read "Parar la aplicación"() -> (w110:bool)
      }
      n870 = case shown="True" w83 {
        frame False {
        }
        frame True {
          w91 = T13 {"IP"="169.254.1.1", "Port"=5084, "ReaderConfigFile"=path "", "ROspecConfigFile"=path ""}  # RFID Configuration
          w95 = path "" ("ReaderConfigFile")
          # "Loop RFID reader"
          n871 = local read "Puerto RFID"() -> (w93:u16)
          n872 = local read "IP RFID"() -> (w94:string)
          n873 = Bundle By Name(cluster=w91, "IP"=w94, "Port"=w93, "ReaderConfigFile"=w95, "ROspecConfigFile"=w95) -> (w92:T13)
          n874 = while {
            tunnel: w92 -> [w97]
            stop <- w98 stop-if-true
            n875 = local read "Parar la aplicación"() -> (w98:bool)
            n876 = call "IF2_Reader.vi"("Stop"=w98, "RFID Configuration"=w97) -> ("error out"=w99:errorcluster, "connection ID"=→"connection ID":refnum<k5>)  [unwired: 8 in]
            n877 = case shown="Error" w99 {
              tunnel: w99 -> [_ w101]
              tunnel: [TRUE ("RFIDStatus") FALSE ("RFIDStatus")] -> _
              frame No Error {
              }
              frame Error {
                n878 = call "Reporting_error.vi"("error out 2"=w101, "Concept"="Passive RFID") -> ("Reporting"=w103:string)  [unwired: 1 in]
                n879 = local read "Report"() -> (w104:string)
                n880 = Concatenate Strings(w103, w104) -> (w102:string)
                n881 = local write "Report"(w102) -> ()
              }
            }
          }
        }
      }
      n882 = xnode "Close FPGA VI Reference"("FPGA VI Reference In"=w86, "error in"=w85) -> ("error out"=→"error FPGA":errorcluster)
    }
    frame #3 {
      n883 = call "LH6HD.vi"("Action"=enum16{"Init", "Start", "Read", "Stop", "Exit"}."Stop") -> ("error out"=→"RFID_LR6_Error":errorcluster)  [unwired: 9 in, 1 out]
    }
  }
